vi "UDS Diagnostics Engine.vi"(8 "error in (no error)":errorcluster, 11 "State Variables":T1={"TCP Refs"={"Connection List"=refnum, "listener ID"=refnum}, "Stop"=refnum, "Top VI"=refnum, "Parameters"={"Properties"={"Name"="", "CAN"={"Database File"=path "", "CAN Interface"=enum."CAN0", "Baud Rate"=0, "Diagnostic Protocol"=enum."GMLAN", "Transport Protocol"=enum."ISO TP - Normal Mode", "Transmit ID"=0, "Receive ID"=0, "Transmit Extension"=0, "Receive Extension"=0, "Receive UUDT ID"=0, "Enable Stream"=TRUE, "VW TP Channel ID"=0, "Security"={"Source DLL Path"=path "", "Security Level"=1, "Target DLL Path"=path ""}, "Fill Frame"=FALSE, "Fill Byte"=255, "Termination"=FALSE}, "FPGA Settings"={"RT Bitfile Path"=path "", "RIO Device"=0, "Enable"=FALSE}, "PIDs"=[], "PID Lookup"=variant, "CPIDs"=[], "CPID Lookup"=variant, "DIDs"=[], "DID Lookup"=variant, "DPIDs"=[], "DPID Lookup"=variant, "DTC descriptor"={"DTC Byte Length"=2, "Status Byte Length"=1, "Add Data Byte Length"=1, "Byte Order"=enum."Motorola"}, "Routines"=[], "Routine Lookups"={"Start.Cmd"=variant, "Start.Resp"=variant, "Status.Cmd"=variant, "Status.Resp"=variant, "Stop.Cmd"=variant, "Stop.Resp"=variant}, "IO Control"=[], "IO.Cmd Lookup"=variant, "IO.Resp Lookup"=variant, "Memory Writes"=[], "Memory.Write Lookup"=variant, "Memory Reads"=[], "Memory.Read Lookup"=variant, "DTCControl"={"Description"="", "Signals"=[]}}, "ChanRefs"={"ToVS.PIDs"={"Name"="", "Write to VS Engine FIFO"=refnum, "Pairs"={"Refs"=[], "Values"=[]}}, "ToVS.DIDs"={"Name"="", "Write to VS Engine FIFO"=refnum, "Pairs"={"Refs"=[], "Values"=[]}}, "ToVS.DTCs"={"Name"="", "Write to VS Engine FIFO"=refnum, "Pairs"={"Refs"=[], "Values"=[]}}, "ToVS.DTCCount"={"Name"="", "Write to VS Engine FIFO"=refnum, "Pairs"={"Refs"=[], "Values"=[]}}, "ToVS.Status"={"Name"="", "Write to VS Engine FIFO"=refnum, "Pairs"={"Refs"=[], "Values"=[]}}, "FromVS.CPIDs"={"Name"="", "Read from VS Engine FIFO"=refnum, "Pairs"={"Refs"=[], "Values"=[]}}, "Cmds"={"Name"="", "Write to VS Engine FIFO"=refnum, "Read from VS Engine FIFO"=refnum, "Pairs"={"Chan Refs"=[], "Prev. Values"=[]}}, "FromVS.Routine.Start"={"Name"="", "Read from VS Engine FIFO"=refnum, "Pairs"={"Refs"=[], "Values"=[]}}, "ToVS.Routine.Start"={"Name"="", "Write to VS Engine FIFO"=refnum, "Pairs"={"Refs"=[], "Values"=[]}}, "FromVS.Routine.Status"={"Name"="", "Read from VS Engine FIFO"=refnum, "Pairs"={"Refs"=[], "Values"=[]}}, "ToVS.Routine.Status"={"Name"="", "Write to VS Engine FIFO"=refnum, "Pairs"={"Refs"=[], "Values"=[]}}, "FromVS.Routine.Stop"={"Name"="", "Read from VS Engine FIFO"=refnum, "Pairs"={"Refs"=[], "Values"=[]}}, "ToVS.Routine.Stop"={"Name"="", "Write to VS Engine FIFO"=refnum, "Pairs"={"Refs"=[], "Values"=[]}}, "FromVS.IO.Cmd"={"Name"="", "Read from VS Engine FIFO"=refnum, "Pairs"={"Refs"=[], "Values"=[]}}, "ToVS.IO.Resp"={"Name"="", "Write to VS Engine FIFO"=refnum, "Pairs"={"Refs"=[], "Values"=[]}}, "FromVS.WriteMemory"={"Name"="", "Read from VS Engine FIFO"=refnum, "Pairs"={"Refs"=[], "Values"=[]}}, "ToVS.ReadMemory"={"Name"="", "Write to VS Engine FIFO"=refnum, "Pairs"={"Refs"=[], "Values"=[]}}, "FromVS.DTCControl"={"Name"="", "Read from VS Engine FIFO"=refnum, "Pairs"={"Refs"=[], "Values"=[]}}}}, "ADCS Connection"={"Diag CAN Handle"=0, "Transport Protocol"=enum."ISO TP - Normal Mode", "Receive Address Extension"=0, "Transmit Address Extension"=0, "Receive CAN Id"=0, "Transmit CAN Id"=0, "Diag CAN Queue"=refnum, "Log Frames ?"=FALSE, "My TP Address"=0, "Other TP Address"=0, "T1"=0, "T2"=0, "T3"=0, "T4"=0, "Tx SN"=0, "Block Size"=0, "Rx SN"=0, "VW TP Initialized?"=FALSE, "Tx block no"=0, "baud rate"=0, "Interface"="", "Channel Diag CAN Handle"=0, "UDP Connection ID"=refnum, "TCP Connection ID"=refnum, "Target IP Addr"=0, "Source Address"=0, "Target Address"=0, "Send Header NACK?"=FALSE, "DLL Handle"=0, "NAD"=0, "Time Stamp read first"=0.0, "Time Stamp read last"=0.0, "Time Stamp write first"=0.0, "Time Stamp write last"=0.0, "Time Stamp write"=0.0, "Time Stamp read"=0.0}, "XNET References"={"Database"="", "GMLAN DPID Session"="", "Cluster"=""}, "BufferedCmds"=refnum, "XNETEngine (GMLAN)"=refnum} {"Parameters"."ChanRefs"."ToVS.ReadMemory"."Pairs"."Refs" format="%.0x"; "Parameters"."ChanRefs"."ToVS.IO.Resp"."Pairs"."Refs" format="%.0x"; "Parameters"."ChanRefs"."ToVS.Routine.Status"."Pairs"."Refs" format="%.0x"; "Parameters"."ChanRefs"."ToVS.Routine.Stop"."Pairs"."Refs" format="%.0x"; "Parameters"."ChanRefs"."ToVS.Routine.Start"."Pairs"."Refs" format="%.0x"; "Parameters"."ChanRefs"."Cmds"."Pairs"."Chan Refs" format="%.0x"; "Parameters"."ChanRefs"."ToVS.Status"."Pairs"."Refs" format="%.0x"; "Parameters"."ChanRefs"."ToVS.DTCCount"."Pairs"."Refs" format="%.0x"; "Parameters"."ChanRefs"."ToVS.DTCs"."Pairs"."Refs" format="%.0x"; "Parameters"."ChanRefs"."ToVS.PIDs"."Pairs"."Refs" format="%.0x"; "Parameters"."ChanRefs"."ToVS.DIDs"."Pairs"."Refs" format="%.0x"; "Parameters"."Properties"."DTCControl"."Signals"."Byte Order" items=["Little Endian", "Big Endian"]; "Parameters"."Properties"."DTCControl"."Signals"."Data Type" items=["Signed", "Unsigned", "IEEE Float"]; "Parameters"."Properties"."Memory Reads"."Signals"."Byte Order" items=["Little Endian", "Big Endian"]; "Parameters"."Properties"."Memory Reads"."Signals"."Data Type" items=["Signed", "Unsigned", "IEEE Float"]; "Parameters"."Properties"."Memory Writes"."Signals"."Byte Order" items=["Little Endian", "Big Endian"]; "Parameters"."Properties"."Memory Writes"."Signals"."Data Type" items=["Signed", "Unsigned", "IEEE Float"]; "Parameters"."Properties"."CPIDs"."Signals"."Byte Order" items=["Little Endian", "Big Endian"]; "Parameters"."Properties"."CPIDs"."Signals"."Data Type" items=["Signed", "Unsigned", "IEEE Float"]; "Parameters"."Properties"."DIDs"."Signals"."Byte Order" items=["Little Endian", "Big Endian"]; "Parameters"."Properties"."DIDs"."Signals"."Data Type" items=["Signed", "Unsigned", "IEEE Float"]; "Parameters"."Properties"."CAN"."Fill Byte" format="%.0x"; "Parameters"."Properties"."CAN"."VW TP Channel ID" format="%.0x"; "Parameters"."Properties"."CAN"."Receive UUDT ID" format="%.0x"; "Parameters"."Properties"."CAN"."Receive Extension" format="%.0x"; "Parameters"."Properties"."CAN"."Transmit Extension" format="%.0x"; "Parameters"."Properties"."CAN"."Receive ID" format="%.0x"; "Parameters"."Properties"."CAN"."Transmit ID" format="%.0x"; "Parameters"."Properties"."PIDs"."Signals"."Byte Order" items=["Little Endian", "Big Endian"]; "Parameters"."Properties"."PIDs"."Signals"."Data Type" items=["Signed", "Unsigned", "IEEE Float"]}) -> (0 "error out":errorcluster)   [LabVIEW 2015, in "Diagnostics Addon Engine.lvlib"]
doc: "Async loop that handles the UDS commands sent either by the channel engine or the TCP engine"
uses:
  Diagnostics Addon Engine.lvlib
  Stop FG/Stop Global Commands.ctl
  Stop FG/Stop FG.lvlib
  Error Handling API/Error Handling API.lvlib
  <vilib>/NI Veristand/Custom Device Tools/Custom Device Utility Library/Custom Device Utility Library.lvlib
  Shared/SubVIs/GUID Lookup.vi
  Shared/Diagnostics Addon Shared.lvlib
  Shared/Types/DTC and Timestamp Cluster.ctl
  Shared/Types/Datatable Lookup Positions.ctl
  <vilib>/NI/AMC/AMC.lvlib
  <vilib>/NI/Tools/Keyed Array/Tools_KeyedArray.lvlib
  GMLAN/GMLAN.lvlib
  GMLAN/_SubVIs/InitiateDiagnosticOperation_Parameter.ctl
  GMLAN/_SubVIs/InitiateDiagnosticOperation_SubFunctions.ctl
  GMLAN/_SubVIs/DisableNormalCommunication_Parameter.ctl
  GMLAN/_SubVIs/ReadDataByPacketIdentifier_SubFunctions.ctl
  <vilib>/Automotive Diagnostic Command Set/Diagnostic Transport.llb/Property ID.ctl
  <vilib>/addons/Automotive Diagnostic Command Set/NI_Automotive Diagnostic Command Set.lvlib
  Types/PID Data.ctl
  Shared/Types/ReadDTCbyDTCNumber Parameters.ctl
  GMLAN/_SubVIs/ReadFailureRecordData_readFailureRecordParameters_failureRecordIdentifier.ctl
  <vilib>/xnet/xnet.llb/XNET Convert (Signal to Frame Raw).vi
  <vilib>/xnet/xnet.llb/XNET Convert (Frame Raw to Signal).vi
  Shared/Types/Input Output Cmd Parameters.ctl
  STM/STM Lookup Table Ref.ctl
  Types/TCP Refs.ctl
  Shared/Types/Signal Parameters.ctl
  Shared/Types/Frame Parameters.ctl
  <vilib>/Automotive Diagnostic Command Set/Diagnostic Protocols.llb/DTC Descriptor.ctl
  Shared/Types/DPID Periodic Rate.ctl
  Shared/Types/DPID Parameters.ctl
  Shared/Types/Diagnostic Protocols.ctl
  Shared/Types/CAN Interface.ctl
  Shared/Types/CAN Configuration.ctl
  Shared/Types/Section Properties.ctl
  Types/Main Configuration.ctl
  Types/XNET References.ctl
  Types/State Variables.ctl
  <vilib>/NI Veristand/Custom Device API/Data Reference.ctl
  <vilib>/NI Veristand/Custom Device API/Custom Device API.lvlib
  Types/VS Data Channels.ctl
  <vilib>/NI Veristand/Custom Device API/Block Data Reference.ctl
  <vilib>/NI/Tools/Keyed Array/KeyedArray.ctl
  <vilib>/NI/AMC/Message.ctl
  <vilib>/NI/AMC/Message Queue.ctl
  Shared/Types/Transport Protocols.ctl
  <vilib>/Automotive Diagnostic Command Set/Diagnostic Transport.llb/Transport Protocol Selector.ctl
  <vilib>/Automotive Diagnostic Command Set/Diagnostic Transport.llb/Diag CAN Frame Log.ctl
  <vilib>/Automotive Diagnostic Command Set/Diagnostic Transport.llb/Diag Reference.ctl
  Inline Async API/Controls/Write To VS Engine.ctl
  Inline Async API/Inline Async API.lvlib
  Inline Async API/Controls/Read From VS Engine.ctl
  Inline Async API/Controls/ReadWrite Data.ctl
  Stop FG/Stop Global Ref.ctl
  Shared/Types/Security.ctl
  Shared/Types/FPGA Bitfile Settings.ctl
  Shared/Types/Command Response Signals.ctl
  Shared/Types/Routine Paramaters.ctl
  Shared/Types/IO Control Parameters.ctl
  Shared/Types/Compiled Routine Lookups.ctl
  Shared/Types/Exported DTC Control Cluster.ctl
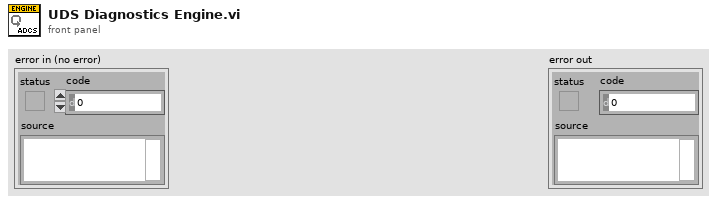
[diagram p1: front panel]
types:
  T1 = typedef "Diagnostics Addon Engine.lvlib/State Variables.ctl" = cluster{"TCP Refs":T2, "Stop":T4, "Top VI":refnum<vi>, "Parameters":T5, "ADCS Connection":T29, "XNET References":T31, "BufferedCmds":T32, "XNETEngine (GMLAN)":T32}
  T2 = typedef "Diagnostics Addon Engine.lvlib/TCP Refs.ctl" = cluster{"Connection List":T3, "listener ID":refnum<k5>}
  T3 = typedef "Diagnostics Addon Engine.lvlib/STM Lookup Table Ref.ctl" = refnum<vi>
  T4 = typedef "Diagnostics Addon Engine.lvlib/Stop FG.lvlib/Stop Global Ref.ctl" = refnum<vi>
  T5 = typedef "Diagnostics Addon Engine.lvlib/Main Configuration.ctl" = cluster{"Properties":T6, "ChanRefs":T23}
  T6 = typedef "Diagnostics Addon Shared.lvlib/Section Properties.ctl" = cluster{"Name":string, "CAN":T7, "FPGA Settings":T12, "PIDs":T13[], "PID Lookup":variant, "CPIDs":T13[], "CPID Lookup":variant, "DIDs":T13[], "DID Lookup":variant, "DPIDs":T15[], "DPID Lookup":variant, "DTC descriptor":T17, "Routines":T18[], "Routine Lookups":T20, "IO Control":T21[], "IO.Cmd Lookup":variant, "IO.Resp Lookup":variant, "Memory Writes":T13[], "Memory.Write Lookup":variant, "Memory Reads":T13[], "Memory.Read Lookup":variant, "DTCControl":T22}
  T7 = typedef "Diagnostics Addon Shared.lvlib/CAN Configuration.ctl" = cluster{"Database File":path, "CAN Interface":T8, "Baud Rate":u32, "Diagnostic Protocol":T9, "Transport Protocol":T10, "Transmit ID":u32, "Receive ID":u32, "Transmit Extension":u8, "Receive Extension":u8, "Receive UUDT ID":u32, "Enable Stream":bool, "VW TP Channel ID":u32, "Security":T11, "Fill Frame":bool, "Fill Byte":u8, "Termination":bool}
  T8 = typedef "Diagnostics Addon Shared.lvlib/CAN Interface.ctl" = enum16{"CAN0", "CAN1", "CAN2", "CAN3", "CAN4", "CAN5", "CAN6", "CAN7", "CAN8", "CAN9", "CAN10", "CAN11", "CAN12", "CAN13", "CAN14", "CAN15", "CAN16", "CAN17", "CAN18", "CAN19", "CAN20", "CAN21", "CAN22", "CAN23", "CAN24", "CAN25", "CAN26", "CAN27", "CAN28", "CAN29", "CAN30", "CAN31", "CAN32", "CAN33", "CAN34", "CAN35", "CAN36", "CAN37", "CAN38", "CAN39", "CAN40", "CAN41", "CAN42", "CAN43", "CAN44", "CAN45", "CAN46", "CAN47", "CAN48", "CAN49", "CAN50", "CAN51", "CAN52", "CAN53", "CAN54", "CAN55", "CAN56", "CAN57", "CAN58", "CAN59", "CAN60", "CAN61", "CAN62", "CAN63", "CAN 256 (Virtual)", "CAN 257 (Virtual)"}
  T9 = typedef "Diagnostics Addon Shared.lvlib/Diagnostic Protocols.ctl" = enum16{"GMLAN", "KWP-2000", "UDS"}
  T10 = typedef "Diagnostics Addon Shared.lvlib/Transport Protocols.ctl" = enum16{"ISO TP - Normal Mode", "ISO TP - Mixed Mode", "VW TP 2.0", "Diagnostics on IP"}
  T11 = typedef "Diagnostics Addon Shared.lvlib/Security.ctl" = cluster{"Source DLL Path":path, "Security Level":u8, "Target DLL Path":path}
  T12 = typedef "Diagnostics Addon Shared.lvlib/FPGA Bitfile Settings.ctl" = cluster{"RT Bitfile Path":path, "RIO Device":u16, "Enable":bool}
  T13 = typedef "Diagnostics Addon Shared.lvlib/Frame Parameters.ctl" = cluster{"Name":string, "Description":string, "ID":u32, "Signals":T14[]}
  T14 = typedef "Diagnostics Addon Shared.lvlib/Signal Parameters.ctl" = cluster{"Start Bit":u8, "Length":u8, "Scaling Factor":dbl, "Scaling Offset":dbl, "Minimum":dbl, "Maximum":dbl, "Data Type":u32, "Byte Order":u32, "Default Value":dbl, "Name":string, "Units":string, "Description":string}
  T15 = typedef "Diagnostics Addon Shared.lvlib/DPID Parameters.ctl" = cluster{"DPID ID":u8, "Speed":T16, "PIDs":u16[]}
  T16 = typedef "Diagnostics Addon Shared.lvlib/DPID Periodic Rate.ctl" = enum16{"Slow", "Medium", "Fast"}
  T17 = typedef "Diagnostics Addon Shared.lvlib/DTC Descriptor.ctl" = cluster{"DTC Byte Length":i32, "Status Byte Length":i32, "Add Data Byte Length":i32, "Byte Order":enum16{"Motorola", "Intel"}}
  T18 = typedef "Diagnostics Addon Shared.lvlib/Routine Paramaters.ctl" = cluster{"Name":string, "Description":string, "ID":u16, "Start Parameters":T19, "Request Parameters":T19, "Stop Parameters":T19}
  T19 = typedef "Diagnostics Addon Shared.lvlib/Command Response Signals.ctl" = cluster{"Cmd":T14[], "Response":T14[]}
  T20 = typedef "Diagnostics Addon Shared.lvlib/Compiled Routine Lookups.ctl" = cluster{"Start.Cmd":variant, "Start.Resp":variant, "Status.Cmd":variant, "Status.Resp":variant, "Stop.Cmd":variant, "Stop.Resp":variant}
  T21 = typedef "Diagnostics Addon Shared.lvlib/IO Control Parameters.ctl" = cluster{"Name":string, "Description":string, "ID":u16, "Signals":T19}
  T22 = typedef "Diagnostics Addon Shared.lvlib/Exported DTC Control Cluster.ctl" = cluster{"Description":string, "Signals":T14[]}
  T23 = typedef "Diagnostics Addon Engine.lvlib/VS Data Channels.ctl" = cluster{"ToVS.PIDs":T24, "ToVS.DIDs":T24, "ToVS.DTCs":T24, "ToVS.DTCCount":T24, "ToVS.Status":T24, "FromVS.CPIDs":T26, "Cmds":T28, "FromVS.Routine.Start":T26, "ToVS.Routine.Start":T24, "FromVS.Routine.Status":T26, "ToVS.Routine.Status":T24, "FromVS.Routine.Stop":T26, "ToVS.Routine.Stop":T24, "FromVS.IO.Cmd":T26, "ToVS.IO.Resp":T24, "FromVS.WriteMemory":T26, "ToVS.ReadMemory":T24, "FromVS.DTCControl":T26}
  T24 = typedef "Diagnostics Addon Engine.lvlib/Inline Async API.lvlib/Write To VS Engine.ctl" = cluster{"Name":string, "Write to VS Engine FIFO":refnum<k33>, "Pairs":cluster{"Refs":T25[], "Values":dbl[]}}
  T25 = typedef "Custom Device API.lvlib/Data Reference.ctl" = i32
  T26 = typedef "Diagnostics Addon Engine.lvlib/Inline Async API.lvlib/Read From VS Engine.ctl" = cluster{"Name":string, "Read from VS Engine FIFO":refnum<k33>, "Pairs":cluster{"Refs":T27[], "Values":dbl[]}}
  T27 = typedef "Custom Device API.lvlib/Block Data Reference.ctl" = cluster{"Data Reference":T25, "Offset":u64, "Length":u64}
  T28 = typedef "Diagnostics Addon Engine.lvlib/Inline Async API.lvlib/ReadWrite Data.ctl" = cluster{"Name":string, "Write to VS Engine FIFO":refnum<k33>, "Read from VS Engine FIFO":refnum<k33>, "Pairs":cluster{"Chan Refs":T25[], "Prev. Values":dbl[]}}
  T29 = typedef "NI_Automotive Diagnostic Command Set.lvlib/Diag Reference.ctl" = cluster{"Diag CAN Handle":u32, "Transport Protocol":T30, "Receive Address Extension":u8, "Transmit Address Extension":u8, "Receive CAN Id":u32, "Transmit CAN Id":u32, "Diag CAN Queue":refnum<queue>, "Log Frames ?":bool, "My TP Address":u8, "Other TP Address":u8, "T1":u16, "T2":u16, "T3":u16, "T4":u16, "Tx SN":u8, "Block Size":u8, "Rx SN":u8, "VW TP Initialized?":bool, "Tx block no":u8, "baud rate":u32, "Interface":string, "Channel Diag CAN Handle":u32, "UDP Connection ID":refnum<k16>, "TCP Connection ID":refnum<k5>, "Target IP Addr":u32, "Source Address":u16, "Target Address":u16, "Send Header NACK?":bool, "DLL Handle":u32, "NAD":u8, "Time Stamp read first":dbl, "Time Stamp read last":dbl, "Time Stamp write first":dbl, "Time Stamp write last":dbl, "Time Stamp write":dbl, "Time Stamp read":dbl}
  T30 = typedef "NI_Automotive Diagnostic Command Set.lvlib/Transport Protocol Selector.ctl" = enum16{"ISO TP - Normal Mode", "ISO TP - Mixed Mode", "VW TP 2.0", "Diagnostics on IP", "ISO TP LIN"}
  T31 = typedef "Diagnostics Addon Engine.lvlib/XNET References.ctl" = cluster{"Database":refnum<k21>, "GMLAN DPID Session":refnum<k21>, "Cluster":refnum<k21>}
  T32 = typedef "AMC.lvlib/Message Queue.ctl" = refnum<queue>
  T33 = typedef "Diagnostics Addon Shared.lvlib/DTC and Timestamp Cluster.ctl" = cluster{"Timestamp":dbl, "DTC":dbl, "Status":dbl, "Add Data":dbl}
  T34 = typedef "Diagnostics Addon Engine.lvlib/Stop FG.lvlib/Stop Global Commands.ctl" = enum16{"Write", "Read", "Reset"}
  T35 = typedef "NI_Automotive Diagnostic Command Set.lvlib/Property ID.ctl" = enum16{"Timeout Diag Command", "Timeout FC (Bs)", "Timeout CF (Cr)", "Receive Block Size (BS)", "Wait Time CF (STmin)", "Max Wait Frames (N_WFTmax)", "Wait Frames to Send (N_WAIT)", "Time between Waits (T_W)", "Fill CAN Frames", "Fill Byte", "Invalid Response as Error", "Max RspPending Count", "VWTP Command Timeout", "STmin", "P2min", "Termination"}
  T36 = typedef "Diagnostics Addon Shared.lvlib/ReadDTCbyDTCNumber Parameters.ctl" = cluster{"DTC":u16, "FailTypeByte":u8}
  T37 = typedef "GMLAN.lvlib/ReadFailureRecordData_readFailureRecordParameters_failureRecordIdentifier.ctl" = cluster{"failureRecordNumber":u8, "DTC ID":u16, "DTCFailureType":u8}
  T38 = enum16{"open", "replace", "create", "open or create", "replace or create", "replace or create with confirmation"}
  T39 = typedef "GMLAN.lvlib/ReadDataByPacketIdentifier_SubFunctions.ctl" = enum8{"stopSending", "sendOneResponse", "scheduleAtSlowRate", "scheduleAtMediumRate", "scheduleAtFastRate"}
  T40 = typedef "GMLAN.lvlib/InitiateDiagnosticOperation_Parameter.ctl" = enum8{"SpecificECU", "EntireNetwork"}
  T41 = typedef "GMLAN.lvlib/DisableNormalCommunication_Parameter.ctl" = enum8{"SpecificECU", "EntireNetwork"}
  T42 = typedef "Diagnostics Addon Engine.lvlib/PID Data.ctl" = cluster{"ID":u16, "Raw Frame":u8[]}
  T43 = cluster{"resp":u8[], "error code":u8, "error out":errorcluster}
  T44 = typedef "Diagnostics Addon Shared.lvlib/Datatable Lookup Positions.ctl" = cluster{"Offset":i32, "Length":i32, "ByteLength":u16}
  T45 = typedef "Diagnostics Addon Shared.lvlib/Input Output Cmd Parameters.ctl" = cluster{"ID":u16, "Mode":u8}
  T46 = typedef "AMC.lvlib/Message.ctl" = cluster{"name":string, "value":string, "attributes":T47, "receiver host":string, "receiver process":string, "source host":string, "source process":string, "priority message":bool, "acknowledge message":bool}
  T47 = typedef "Tools_KeyedArray.lvlib/KeyedArray.ctl" = cluster{"keys":string[], "values":string[]}
  T48 = cluster{"Boolean array[0]":bool, "Boolean array[1]":bool, "Boolean array[2]":bool, "Boolean array[3]":bool, "Boolean array[4]":bool, "Boolean array[5]":bool, "Boolean array[6]":bool, "Boolean array[7]":bool}
  T49 = typedef "Diagnostics Addon Engine.lvlib/Filtered DPID IDs.ctl" = cluster{"Slow":u8[], "Medium":u8[], "Fast":u8[]}
  T50 = typedef "GMLAN.lvlib/InitiateDiagnosticOperation_SubFunctions.ctl" = u8
  T51 = typedef "Diagnostic Trouble Code.ctl" = cluster{"DTC":u32, "Status":u32, "Add Data":u32}
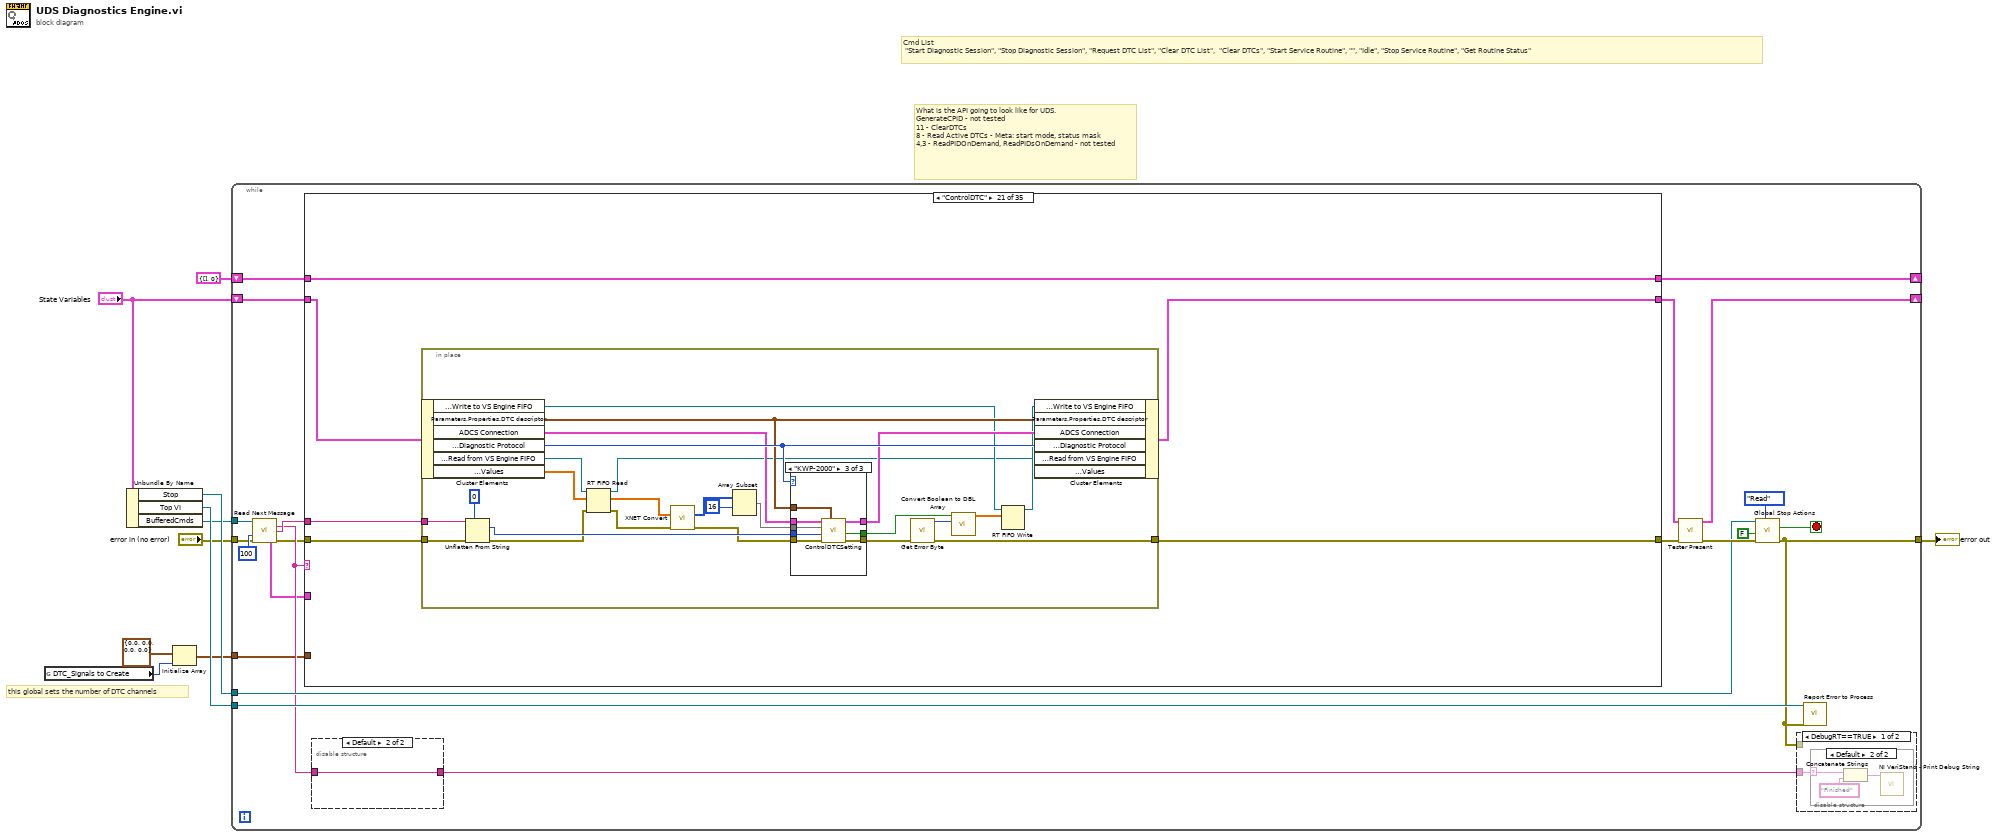
[diagram p0: block diagram]
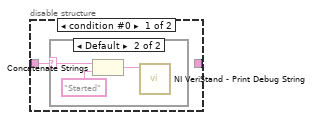
[diagram p2: hidden frame]
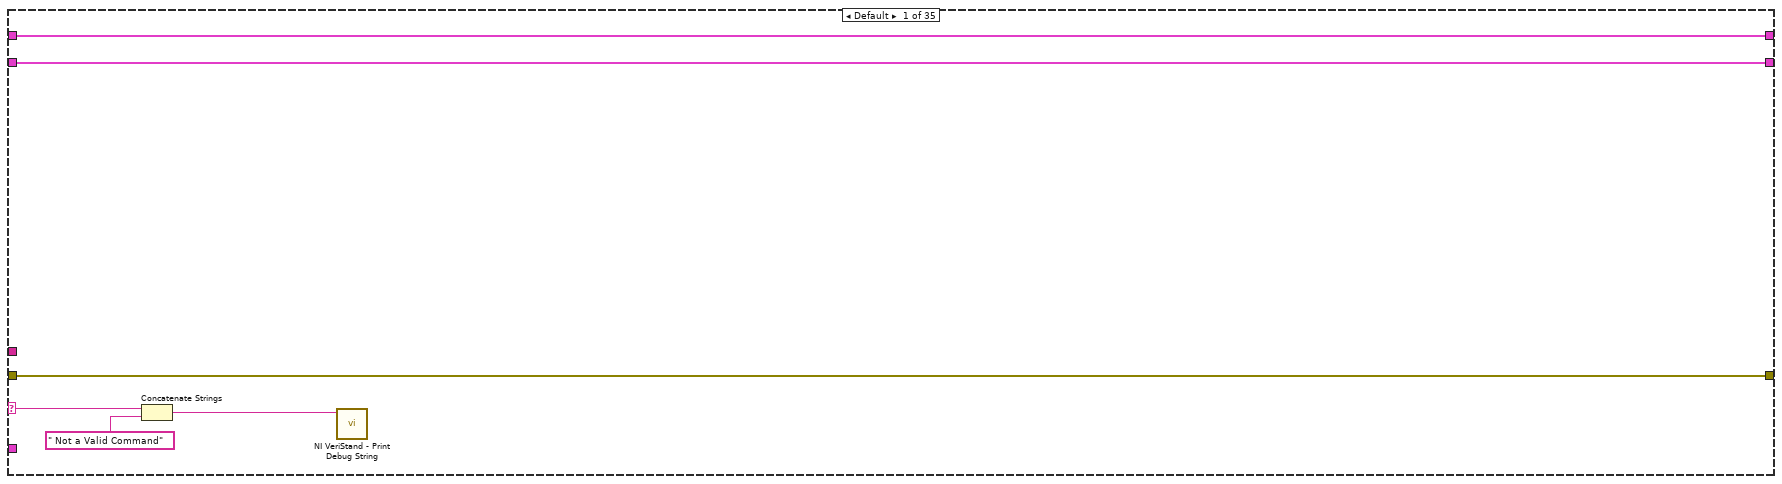
[diagram p6: hidden frame]
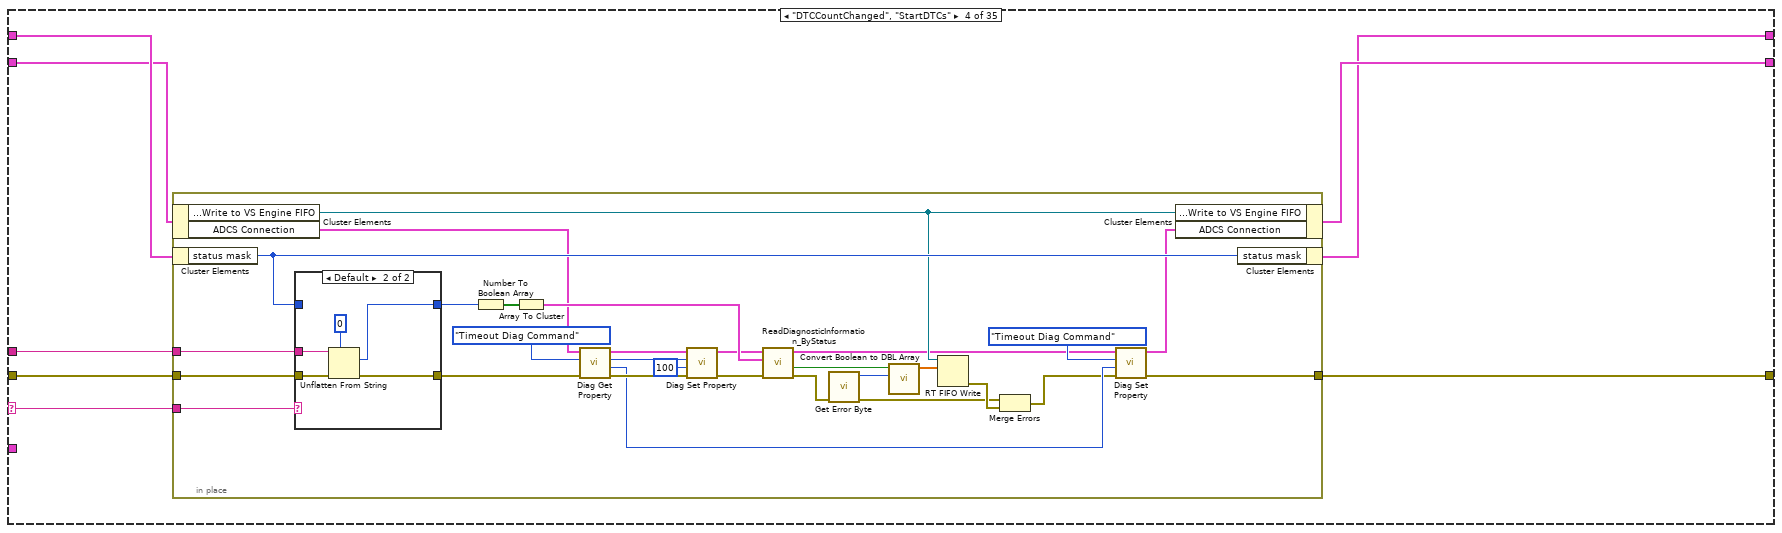
[diagram p9: hidden frame]
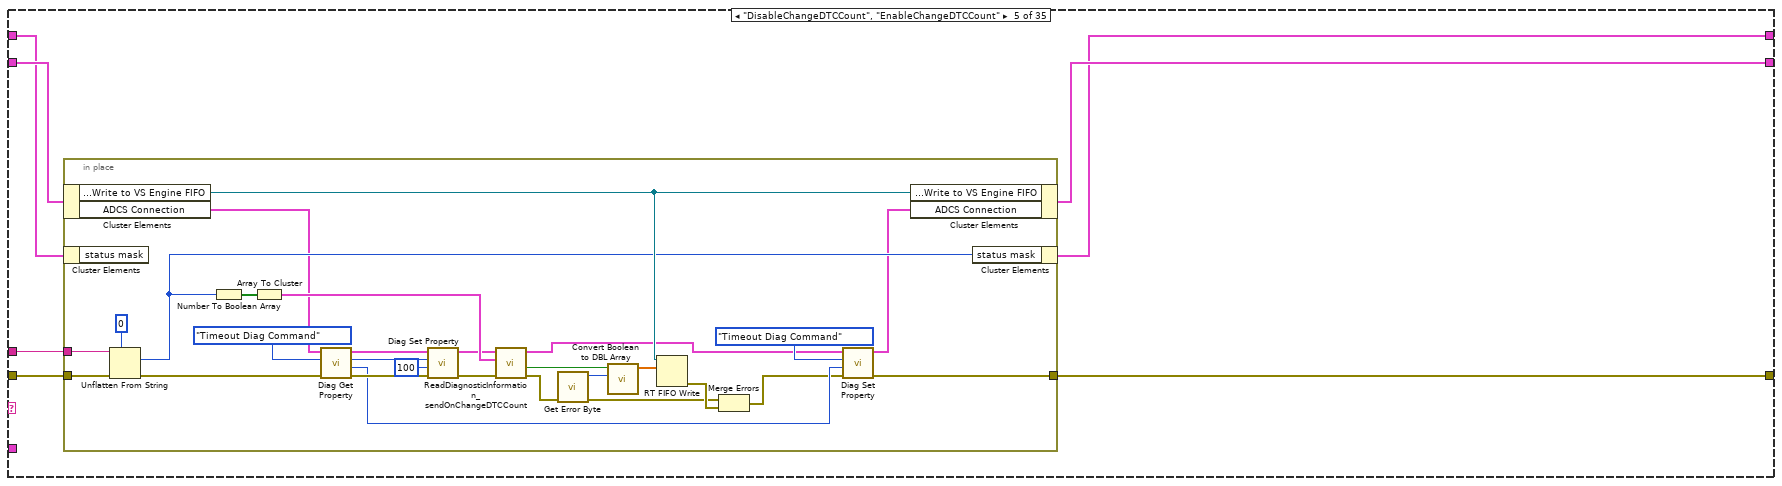
[diagram p11: hidden frame]
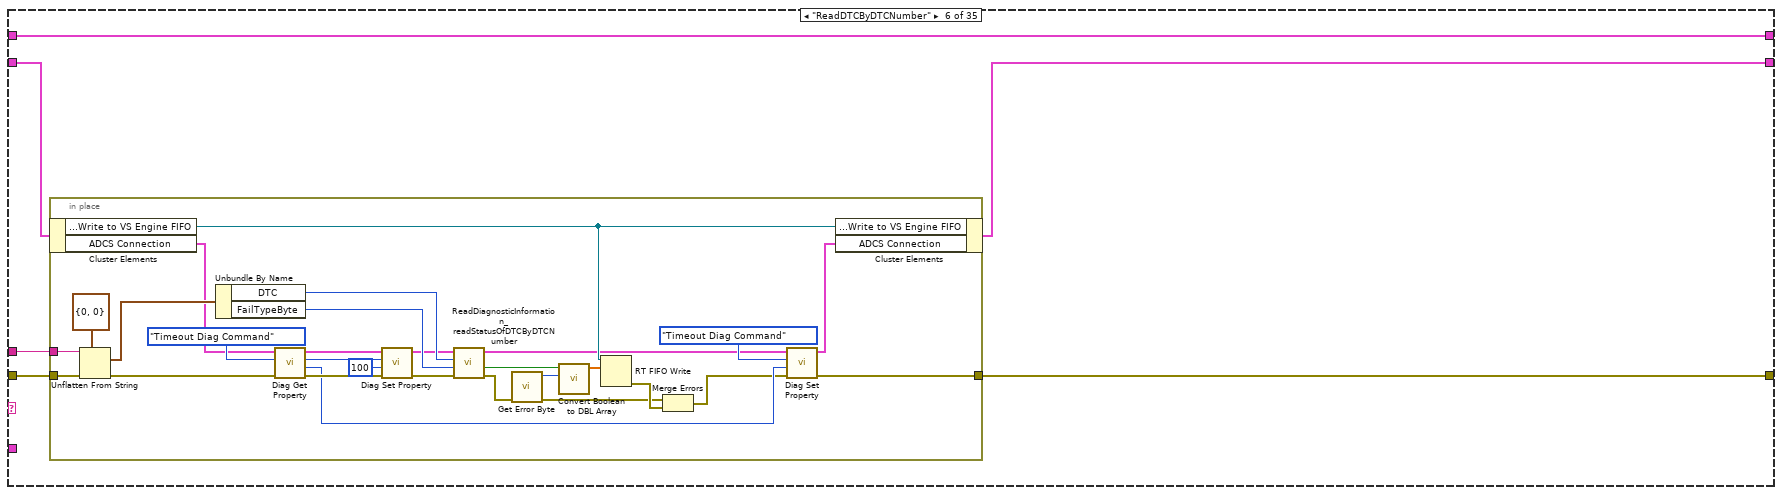
[diagram p12: hidden frame]
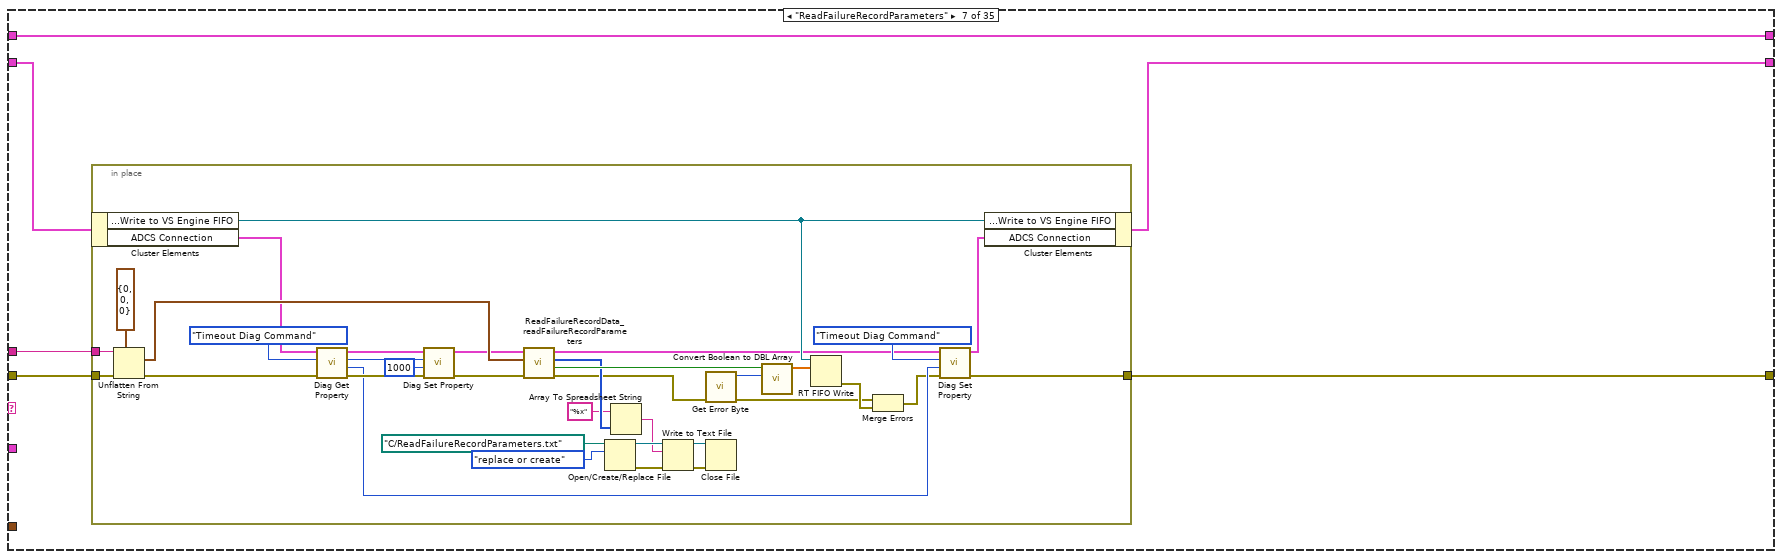
[diagram p13: hidden frame]
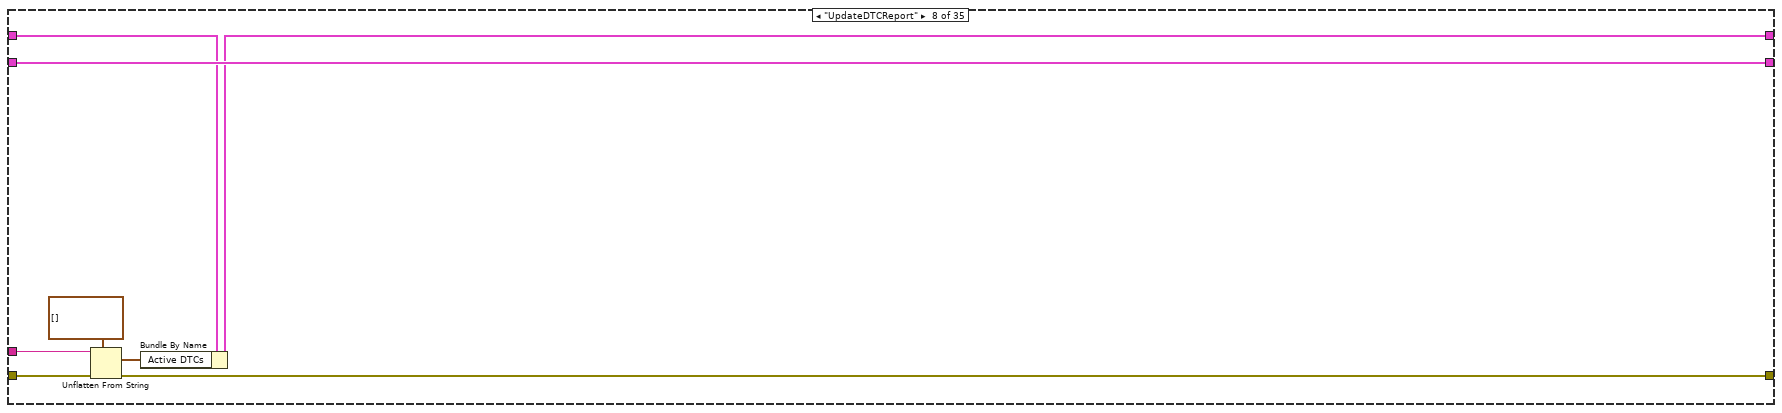
[diagram p14: hidden frame]
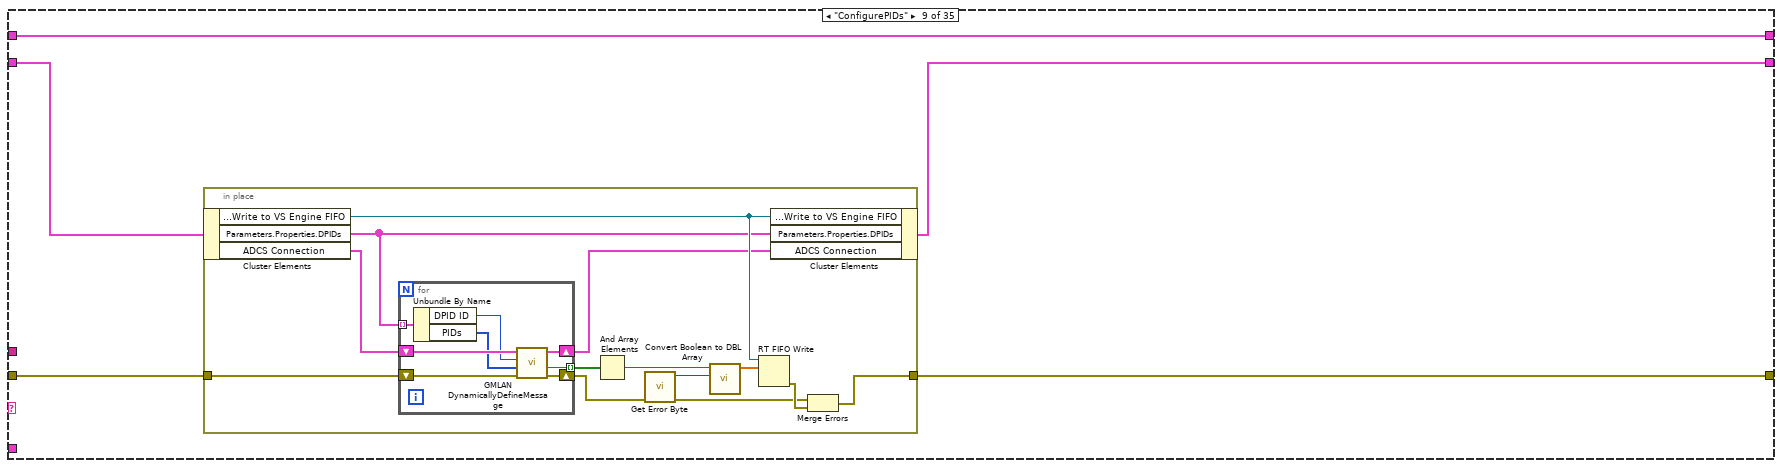
[diagram p15: hidden frame]
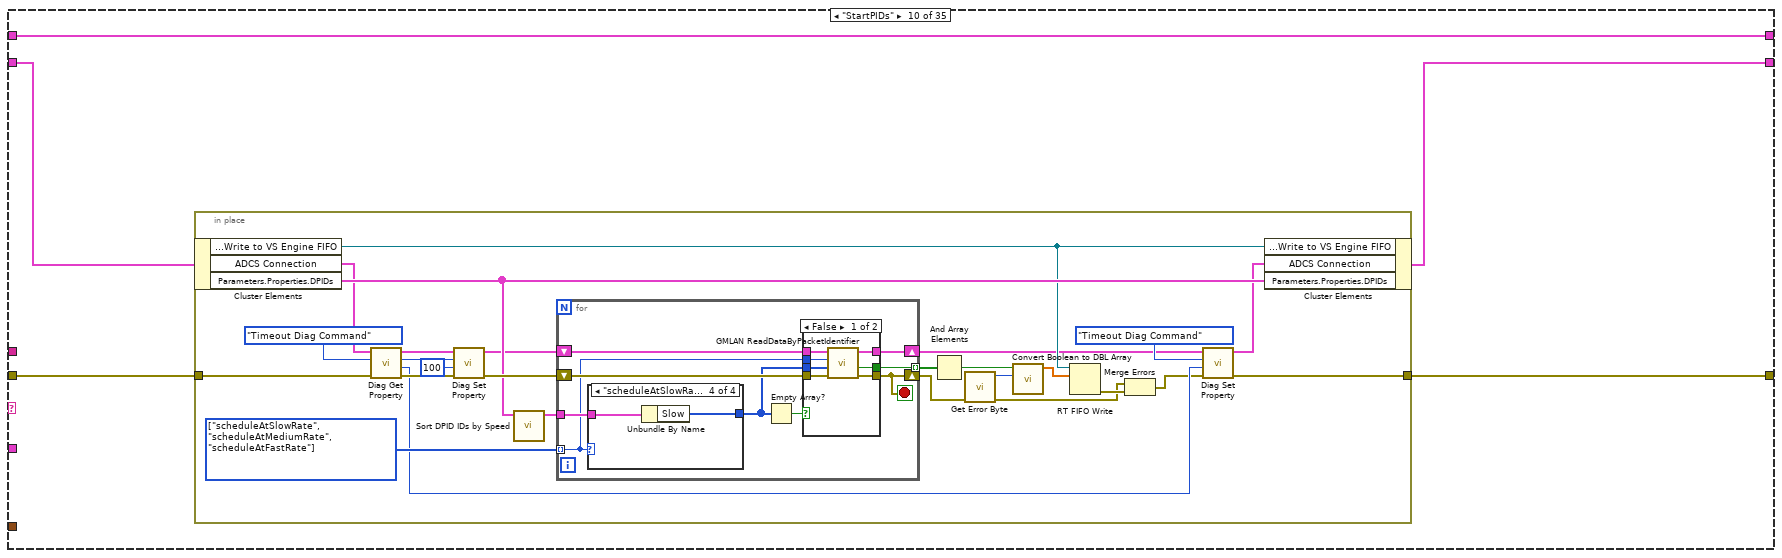
[diagram p16: hidden frame]
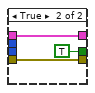
[diagram p17: hidden frame]
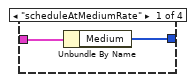
[diagram p18: hidden frame]
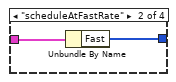
[diagram p19: hidden frame]
diagram:
  # "this global sets the number of DTC channels"
  # "What is the API going to look like for UDS.\nGenerateCPID - not tested\n11 - ClearDTCs\n8 - Read Active DTCs - Meta: start mode, status mask \n4,3 - ReadPIDOnDemand, ReadPIDsOnDemand - not tested"
  # "Cmd List\n \"Start Diagnostic Session\", \"Stop Diagnostic Session\", \"Request DTC List\", \"Clear DTC List\",  \"Clear DTCs\", \"Start Service Routine\", \"\", \"Idle\", \"Stop Service Routine\", \"Get Routine Status\""
  n1 = global read "GUID Lookup.vi" "DTC_Signals to Create"() -> (w3:i32)
  n2 = Unbundle By Name("State Variables") -> ("Stop"=w10:T4, "Top VI"=w9:refnum<vi>, "BufferedCmds"=w5:T32)
  n3 = Initialize Array(T33 {"Timestamp"=0.0, "DTC"=0.0, "Status"=0.0, "Add Data"=0.0} ("Diagnostic Trouble Code"), w3) -> (w2:T33[])
  n4 = while {
    tunnel: w5 -> [w32]
    tunnel: w9 -> [w24]
    tunnel: "error in (no error)" -> [w30]
    tunnel: [w11] -> w8
    tunnel: w10 -> [w23]
    shift-right: [w22] -> _
    shift-left: cluster{"Active DTCs":T33[], "status mask":u8} {"Active DTCs"=[], "status mask"=0} -> [w21]
    tunnel: w2 -> [w18]
    shift-right: [w15] -> _
    shift-left: "State Variables" -> [w17]
    stop <- w25 stop-if-true
    n5 = call <vilib>:"Read Next Message.vi"("message queue in"=w32, "timeout (1 ms)"=100 ("timeout (1ms)"), "error in"=w30) -> ("message name"=w20:string, "message value"=w29:string, "message"=w19:T46, "error out"=w14:errorcluster)  [unwired: 5 in, 4 out]
    n6 = case shown="\"ControlDTC\"" w20 {
      selector: w20 -> [w43 _ _ w59 _ _ _ _ _ _ _ _ _ _ _ _ _ _ _ _ _ w762 _ w971 w1058 _ _ w1149 _ _ _ _ _ _ _]
      tunnel: w14 -> [w47 w50 w51 w61 w103 w134 w167 w208 w215 w239 w296 w335 w338 w344 w358 w398 w434 w471 w508 w530 w711 w759 w870 w973 w1057 w1108 w1142 w1147 w1185 w1192 w1245 w1294 w1419 w1478 w1535]
      tunnel: w29 -> [_ _ _ w58 w101 w135 w168 w204 _ _ _ _ _ _ w356 _ _ _ _ w529 w709 w760 w869 w972 w1056 w1106 _ w1148 _ w1190 w1243 w1293 w1415 w1477 w1534]
      tunnel: [w47 w50 w51 w60 w102 w133 w166 w207 w214 w238 w295 w335 w338 w343 w357 w399 w435 w472 w507 w532 w710 w761 w868 w970 w1055 w1107 w1142 w1150 w1185 w1191 w1244 w1292 w1418 w1476 w1532] -> w12
      tunnel: [w46 w49 w53 w54 w97 w136 w169 w205 w216 w242 w297 w337 w340 w345 w359 w400 w436 w473 w509 w525 w714 _ w871 w974 w1059 w1109 w1144 w1152 w1187 w1193 w1246 w1295 w1420 w1479 w1537] -> w22
      tunnel: w21 -> [w46 w49 w53 w57 w98 w136 w169 w206 w216 w242 w297 w337 w340 w345 w359 w400 w436 w473 w509 w526 w714 _ w871 w974 w1059 w1109 w1144 w1152 w1187 w1193 w1246 w1295 w1420 w1479 w1537]
      tunnel: w19 -> [_ _ _ _ _ _ _ _ _ _ _ _ _ _ _ _ _ _ _ w531 _ w763 _ _ _ _ _ w1151 _ _ _ _ _ _ _]
      tunnel: w18 -> [_ _ _ _ _ _ _ _ _ _ _ _ _ _ _ _ _ _ _ w528 _ _ _ _ _ _ _ _ _ _ _ _ _ _ _]
      tunnel: w17 -> [w42 w48 w52 w56 w100 w132 w165 w211 w213 w241 w294 w336 w339 w342 w355 w397 w433 w470 w506 w527 w713 w758 w867 w969 w1054 w1105 w1143 w1146 w1186 w1189 w1242 w1291 w1417 w1475 w1536]
      tunnel: [w42 w48 w52 w55 w99 w131 w164 w211 w212 w240 w293 w336 w339 w341 w354 w396 w432 w469 w505 w524 w712 w757 w866 w968 w1053 w1104 w1143 w1145 w1186 w1188 w1241 w1290 w1416 w1474 w1533] -> w16
      frame Default {
        n7 = Concatenate Strings(w43, " Not a Valid Command" ("string")) -> (w44:string)
        n8 = call <vilib>:"NI VeriStand - Print Debug String.vi"("Message"=w44) -> ()  [unwired: 10 in, 1 out]
      }
      frame "" {
      }
      frame "<--------------- GMLAN ONLY --------------->" {
      }
      frame "DTCCountChanged", "StartDTCs" {
        n9 = in-place {
          in-place-border: w61 -> [w75]
          in-place-border: [w74] -> w60
          in-place-border: w59 -> [w73]
          in-place-border: w58 -> [w72]
          w87 = Property_ID."Timeout Diag Command" ("property ID")
          n10 = in-place-cluster #1(w56) -> ("Parameters.ChanRefs.ToVS.Status.Write to VS Engine FIFO"=w70:refnum<k33>, "ADCS Connection"=w68:T29)
          n11 = in-place-cluster #2(w57) -> ("status mask"=w71:u8)
          n12 = case shown="Default" w73 {
            tunnel: w75 -> [w91 w96]
            tunnel: w72 -> [_ w95]
            tunnel: [w90 w93] -> w78
            tunnel: [w91 w92] -> w85
            tunnel: w71 -> [w90 _]
            frame "DTCCountChanged" {
            }
            frame Default {
              n13 = Unflatten From String(type=u8 0 ("status mask"), binary string=w95, error in (no error)=w96) -> (value=w93:u8, error out=w92:errorcluster)  [unwired: 2 in, 1 out]
            }
          }
          n14 = Number To Boolean Array(number=w78) -> (Boolean array=w77:bool[])
          n15 = Array To Cluster(array=w77) -> (cluster=w76:T48)
          n16 = call <vilib>:"Diag Get Property.vi"("error in (no error)"=w85, "property ID"=w87, "diag ref in"=w68) -> ("error out"=w89:errorcluster, "property value"=w83:u32, "diag ref out"=w69:T29)  [unwired: 6 in]
          n17 = call <vilib>:"Diag Set Property.vi"("error in (no error)"=w89, "property value"=u32 100, "property ID"=w87, "diag ref in"=w69) -> ("error out"=w84:errorcluster, "diag ref out"=w67:T29)  [unwired: 6 in]
          n18 = call "ReadDiagnosticInformation_ByStatus.vi"("error in (no error)"=w84, "status mask"=w76, "diag ref in"=w67) -> ("error out"=w64:errorcluster, "success?"=w81:bool, "diag ref out"=w66:T29)  [unwired: 5 in, 1 out]
          n19 = call "Get Error Byte.vi"("error"=w64) -> ("error  out"=w63:errorcluster, "Error Byte"=w62:u8)  [unwired: 9 in]
          n20 = call "Convert Boolean to DBL Array.vi"("Error Code"=w62, "Boolean"=w81) -> ("DBL Array"=w82:dbl[])  [unwired: 9 in]
          n21 = RT FIFO Write(0:w70, 1:w82) -> (11:w80:errorcluster)  [unwired: 3 in, 3 out]
          n22 = Merge Errors(w63, w80) -> (w79:errorcluster)
          n23 = call <vilib>:"Diag Set Property.vi"("error in (no error)"=w79, "property value"=w83, "property ID"=Property_ID."Timeout Diag Command", "diag ref in"=w66) -> ("error out"=w74:errorcluster, "diag ref out"=w65:T29)  [unwired: 6 in]
          n24 = in-place-cluster #1("Parameters.ChanRefs.ToVS.Status.Write to VS Engine FIFO"=w70, "ADCS Connection"=w65) -> (w55:T1)
          n25 = in-place-cluster #2("status mask"=w71) -> (w54:cluster{"Active DTCs":T33[], "status mask":u8})
        }
      }
      frame "DisableChangeDTCCount", "EnableChangeDTCCount" {
        n26 = in-place {
          in-place-border: w103 -> [w116]
          in-place-border: [w115] -> w102
          in-place-border: w101 -> [w114]
          w127 = Property_ID."Timeout Diag Command" ("property ID")
          n27 = in-place-cluster #3(w100) -> ("Parameters.ChanRefs.ToVS.Status.Write to VS Engine FIFO"=w113:refnum<k33>, "ADCS Connection"=w110:T29)
          n28 = in-place-cluster #4(w98) -> ()  [unwired: 1 out]
          n29 = Unflatten From String(type=u8 0 ("status mask"), binary string=w114, error in (no error)=w116) -> (value=w112:u8, error out=w125:errorcluster)  [unwired: 2 in, 1 out]
          n30 = Number To Boolean Array(number=w112) -> (Boolean array=w118:bool[])
          n31 = Array To Cluster(array=w118) -> (cluster=w117:T48)
          n32 = call <vilib>:"Diag Get Property.vi"("error in (no error)"=w125, "property ID"=w127, "diag ref in"=w110) -> ("error out"=w129:errorcluster, "property value"=w123:u32, "diag ref out"=w111:T29)  [unwired: 6 in]
          n33 = call <vilib>:"Diag Set Property.vi"("error in (no error)"=w129, "property value"=u32 100, "property ID"=w127, "diag ref in"=w111) -> ("error out"=w124:errorcluster, "diag ref out"=w109:T29)  [unwired: 6 in]
          n34 = call "ReadDiagnosticInformation_sendOnChangeDTCCount.vi"("error in (no error)"=w124, "status mask"=w117, "diag ref in"=w109) -> ("error out"=w106:errorcluster, "success?"=w121:bool, "diag ref out"=w108:T29)  [unwired: 5 in, 1 out]
          n35 = call "Get Error Byte.vi"("error"=w106) -> ("error  out"=w105:errorcluster, "Error Byte"=w104:u8)  [unwired: 9 in]
          n36 = call "Convert Boolean to DBL Array.vi"("Error Code"=w104, "Boolean"=w121) -> ("DBL Array"=w122:dbl[])  [unwired: 9 in]
          n37 = RT FIFO Write(0:w113, 1:w122) -> (11:w120:errorcluster)  [unwired: 3 in, 3 out]
          n38 = Merge Errors(w105, w120) -> (w119:errorcluster)
          n39 = call <vilib>:"Diag Set Property.vi"("error in (no error)"=w119, "property value"=w123, "property ID"=Property_ID."Timeout Diag Command", "diag ref in"=w108) -> ("error out"=w115:errorcluster, "diag ref out"=w107:T29)  [unwired: 6 in]
          n40 = in-place-cluster #3("Parameters.ChanRefs.ToVS.Status.Write to VS Engine FIFO"=w113, "ADCS Connection"=w107) -> (w99:T1)
          n41 = in-place-cluster #4("status mask"=w112) -> (w97:cluster{"Active DTCs":T33[], "status mask":u8})
        }
      }
      frame "ReadDTCByDTCNumber" {
        n42 = in-place {
          in-place-border: w135 -> [w148]
          in-place-border: w134 -> [w147]
          in-place-border: [w145] -> w133
          w161 = Property_ID."Timeout Diag Command" ("property ID")
          n43 = in-place-cluster #5(w132) -> ("Parameters.ChanRefs.ToVS.Status.Write to VS Engine FIFO"=w146:refnum<k33>, "ADCS Connection"=w143:T29)
          n44 = Unflatten From String(type=T36 {"DTC"=0, "FailTypeByte"=0}, binary string=w148, error in (no error)=w147) -> (value=w151:T36, error out=w159:errorcluster)  [unwired: 2 in, 1 out]
          n45 = Unbundle By Name(w151) -> ("DTC"=w150:u16, "FailTypeByte"=w149:u8)
          n46 = call <vilib>:"Diag Get Property.vi"("error in (no error)"=w159, "property ID"=w161, "diag ref in"=w143) -> ("error out"=w163:errorcluster, "property value"=w157:u32, "diag ref out"=w144:T29)  [unwired: 6 in]
          n47 = call <vilib>:"Diag Set Property.vi"("error in (no error)"=w163, "property value"=u32 100, "property ID"=w161, "diag ref in"=w144) -> ("error out"=w158:errorcluster, "diag ref out"=w142:T29)  [unwired: 6 in]
          n48 = call "ReadDiagnosticInformation_readStatusOfDTCByDTCNumber.vi"("error in (no error)"=w158, "FailTypeByte"=w149, "DTC"=w150, "diag ref in"=w142) -> ("error out"=w139:errorcluster, "success?"=w155:bool, "diag ref out"=w141:T29)  [unwired: 4 in, 1 out]
          n49 = call "Get Error Byte.vi"("error"=w139) -> ("error  out"=w138:errorcluster, "Error Byte"=w137:u8)  [unwired: 9 in]
          n50 = call "Convert Boolean to DBL Array.vi"("Error Code"=w137, "Boolean"=w155) -> ("DBL Array"=w156:dbl[])  [unwired: 9 in]
          n51 = RT FIFO Write(0:w146, 1:w156) -> (11:w154:errorcluster)  [unwired: 3 in, 3 out]
          n52 = Merge Errors(w138, w154) -> (w153:errorcluster)
          n53 = call <vilib>:"Diag Set Property.vi"("error in (no error)"=w153, "property value"=w157, "property ID"=Property_ID."Timeout Diag Command", "diag ref in"=w141) -> ("error out"=w145:errorcluster, "diag ref out"=w140:T29)  [unwired: 6 in]
          n54 = in-place-cluster #5("Parameters.ChanRefs.ToVS.Status.Write to VS Engine FIFO"=w146, "ADCS Connection"=w140) -> (w131:T1)
        }
      }
      frame "ReadFailureRecordParameters" {
        n55 = in-place {
          in-place-border: w168 -> [w181]
          in-place-border: w167 -> [w180]
          in-place-border: [w179] -> w166
          w201 = Property_ID."Timeout Diag Command" ("property ID")
          n56 = in-place-cluster #6(w165) -> ("Parameters.ChanRefs.ToVS.Status.Write to VS Engine FIFO"=w178:refnum<k33>, "ADCS Connection"=w176:T29)
          n57 = Unflatten From String(type=T37 {"failureRecordNumber"=0, "DTC ID"=0, "DTCFailureType"=0} ("failureRecordIdentifier"), binary string=w181, error in (no error)=w180) -> (value=w182:T37, error out=w199:errorcluster)  [unwired: 2 in, 1 out]
          n58 = call <vilib>:"Diag Get Property.vi"("error in (no error)"=w199, "property ID"=w201, "diag ref in"=w176) -> ("error out"=w203:errorcluster, "property value"=w197:u32, "diag ref out"=w177:T29)  [unwired: 6 in]
          n59 = call <vilib>:"Diag Set Property.vi"("error in (no error)"=w203, "property value"=u32 1000, "property ID"=w201, "diag ref in"=w177) -> ("error out"=w198:errorcluster, "diag ref out"=w175:T29)  [unwired: 6 in]
          n60 = call "ReadFailureRecordData_readFailureRecordParameters.vi"("error in (no error)"=w198, "failureRecordIdentifier"=w182, "diag ref in"=w175) -> ("error out"=w172:errorcluster, "success?"=w195:bool, "data out"=w188:u8[], "diag ref out"=w174:T29)  [unwired: 5 in]
          n61 = Open/Create/Replace File(file path (use dialog)=path "C:/ReadFailureRecordParameters.txt", operation (0:open)=T38."replace or create") -> (refnum out=w186:refnum<file>, error out=w190:errorcluster)  [unwired: 4 in, 1 out]
          n62 = Array To Spreadsheet String(array=w188, 3:"%x" ("format string")) -> (spreadsheet string=w184:string)  [unwired: 1 in]
          n63 = Write to Text File(file (use dialog)=w186, text=w184, error in=w190) -> (refnum out=w185:refnum<file>, error out=w189:errorcluster)  [unwired: 1 in, 1 out]
          n64 = call "Get Error Byte.vi"("error"=w172) -> ("error  out"=w171:errorcluster, "Error Byte"=w170:u8)  [unwired: 9 in]
          n65 = Close File(refnum=w185, error in=w189) -> ()  [unwired: 2 out]
          n66 = call "Convert Boolean to DBL Array.vi"("Error Code"=w170, "Boolean"=w195) -> ("DBL Array"=w196:dbl[])  [unwired: 9 in]
          n67 = RT FIFO Write(0:w178, 1:w196) -> (11:w194:errorcluster)  [unwired: 3 in, 3 out]
          n68 = Merge Errors(w171, w194) -> (w193:errorcluster)
          n69 = call <vilib>:"Diag Set Property.vi"("error in (no error)"=w193, "property value"=w197, "property ID"=Property_ID."Timeout Diag Command", "diag ref in"=w174) -> ("error out"=w179:errorcluster, "diag ref out"=w173:T29)  [unwired: 6 in]
          n70 = in-place-cluster #6("Parameters.ChanRefs.ToVS.Status.Write to VS Engine FIFO"=w178, "ADCS Connection"=w173) -> (w164:T1)
        }
      }
      frame "UpdateDTCReport" {
        n71 = Unflatten From String(type=T33[] [] ("Active DTCs"), binary string=w204, error in (no error)=w208) -> (value=w210:T33[], error out=w207:errorcluster)  [unwired: 2 in, 1 out]
        n72 = Bundle By Name(cluster=w206, "Active DTCs"=w210) -> (w205:cluster{"Active DTCs":T33[], "status mask":u8})
      }
      frame "ConfigurePIDs" {
        n73 = in-place {
          in-place-border: w215 -> [w229]
          in-place-border: [w224] -> w214
          n74 = in-place-cluster #7(w213) -> ("Parameters.ChanRefs.ToVS.Status.Write to VS Engine FIFO"=w223:refnum<k33>, "Parameters.Properties.DPIDs"=w222:T15[], "ADCS Connection"=w221:T29)
          n75 = for {
            shift-right: [w236] -> w220
            shift-left: w221 -> [w237]
            tunnel: w222 -> [w235] mode=indexing
            shift-right: [w231] -> w219
            shift-left: w229 -> [w232]
            tunnel: [w230] -> w228 mode=indexing
            n76 = Unbundle By Name(w235) -> ("DPID ID"=w234:u8, "PIDs"=w233:u16[])
            n77 = call "GMLAN DynamicallyDefineMessage.vi"("error in (no error)"=w232, "PID List"=w233, "DPID ID"=w234, "diag ref in"=w237) -> ("error out"=w231:errorcluster, "success?"=w230:bool, "diag ref out"=w236:T29)  [unwired: 5 in]
          }
          n78 = And Array Elements(Boolean array=w228) -> (logical AND=w227:bool)
          n79 = call "Get Error Byte.vi"("error"=w219) -> ("error  out"=w218:errorcluster, "Error Byte"=w217:u8)  [unwired: 9 in]
          n80 = call "Convert Boolean to DBL Array.vi"("Error Code"=w217, "Boolean"=w227) -> ("DBL Array"=w226:dbl[])  [unwired: 9 in]
          n81 = RT FIFO Write(0:w223, 1:w226) -> (11:w225:errorcluster)  [unwired: 3 in, 3 out]
          n82 = in-place-cluster #7("Parameters.ChanRefs.ToVS.Status.Write to VS Engine FIFO"=w223, "Parameters.Properties.DPIDs"=w222, "ADCS Connection"=w220) -> (w212:T1)
          n83 = Merge Errors(w218, w225) -> (w224:errorcluster)
        }
      }
      frame "StartPIDs" {
        n84 = in-place {
          in-place-border: w239 -> [w261]
          in-place-border: [w259] -> w238
          w263 = Property_ID."Timeout Diag Command" ("property ID")
          w267 = T39[] [enum."scheduleAtSlowRate", enum."scheduleAtMediumRate", enum."scheduleAtFastRate"] items=["stopSending", "sendOneResponse", "scheduleAtSlowRate", "scheduleAtMediumRate", "scheduleAtFastRate"]
          n85 = in-place-cluster #8(w241) -> ("Parameters.ChanRefs.ToVS.Status.Write to VS Engine FIFO"=w251:refnum<k33>, "ADCS Connection"=w249:T29, "Parameters.Properties.DPIDs"=w252:T15[])
          n86 = call <vilib>:"Diag Get Property.vi"("error in (no error)"=w261, "property ID"=w263, "diag ref in"=w249) -> ("error out"=w265:errorcluster, "property value"=w258:u32, "diag ref out"=w250:T29)  [unwired: 6 in]
          n87 = call <vilib>:"Diag Set Property.vi"("error in (no error)"=w265, "property value"=u32 100, "property ID"=w263, "diag ref in"=w250) -> ("error out"=w260:errorcluster, "diag ref out"=w248:T29)  [unwired: 6 in]
          n88 = call "Sort DPID IDs by Speed.vi"("DPIDs"=w252) -> ("Filtered DPIDs IDs"=w266:T49)  [unwired: 10 in]
          n89 = for {
            tunnel: w266 -> [w273]
            shift-right: [w268] -> w245
            shift-left: w260 -> [w276]
            shift-right: [w274] -> w247
            shift-left: w248 -> [w275]
            tunnel: w267 -> [w270] mode=indexing
            tunnel: [w269] -> w255 mode=indexing
            stop <- w268 stop-if-true
            n90 = case shown="\"scheduleAtSlowRate\"" w270 {
              tunnel: w273 -> [w288 w290 _ w292]
              tunnel: [w287 w289 _ w291] -> w272
              frame "scheduleAtMediumRate" {
                n91 = Unbundle By Name(w288) -> ("Medium"=w287:u8[])
              }
              frame "scheduleAtFastRate" {
                n92 = Unbundle By Name(w290) -> ("Fast"=w289:u8[])
              }
              frame Default {
              }
              frame "scheduleAtSlowRate" {
                n93 = Unbundle By Name(w292) -> ("Slow"=w291:u8[])
              }
            }
            n94 = Empty Array?(array=w272) -> (empty?=w271:bool)
            n95 = case shown="False" w271 {
              tunnel: w276 -> [w283 w285]
              tunnel: [w282 w285] -> w268
              tunnel: w275 -> [w281 w286]
              tunnel: [w280 w286] -> w274
              tunnel: w270 -> [w277 _]
              tunnel: w272 -> [w279 _]
              tunnel: [w278 TRUE ("success?")] -> w269
              frame False {
                n96 = call "GMLAN ReadDataByPacketIdentifier.vi"("error in (no error)"=w283, "DPIDs"=w279, "Sub Function"=w277, "diag ref in"=w281) -> ("error out"=w282:errorcluster, "success?"=w278:bool, "diag ref out"=w280:T29)  [unwired: 4 in, 1 out]
              }
              frame True {
              }
            }
          }
          n97 = And Array Elements(Boolean array=w255) -> (logical AND=w257:bool)
          n98 = call "Get Error Byte.vi"("error"=w245) -> ("error  out"=w244:errorcluster, "Error Byte"=w243:u8)  [unwired: 9 in]
          n99 = call "Convert Boolean to DBL Array.vi"("Error Code"=w243, "Boolean"=w257) -> ("DBL Array"=w256:dbl[])  [unwired: 9 in]
          n100 = RT FIFO Write(0:w251, 1:w256) -> (11:w254:errorcluster)  [unwired: 3 in, 3 out]
          n101 = Merge Errors(w244, w254) -> (w253:errorcluster)
          n102 = call <vilib>:"Diag Set Property.vi"("error in (no error)"=w253, "property value"=w258, "property ID"=Property_ID."Timeout Diag Command", "diag ref in"=w247) -> ("error out"=w259:errorcluster, "diag ref out"=w246:T29)  [unwired: 6 in]
          n103 = in-place-cluster #8("Parameters.ChanRefs.ToVS.Status.Write to VS Engine FIFO"=w251, "ADCS Connection"=w246, "Parameters.Properties.DPIDs"=w252) -> (w240:T1)
        }
      }
      frame "StopPIDs" {
        n104 = in-place {
          in-place-border: w296 -> [w318]
          in-place-border: [w316] -> w295
          w320 = Property_ID."Timeout Diag Command" ("property ID")
          n105 = in-place-cluster #9(w294) -> ("Parameters.ChanRefs.ToVS.Status.Write to VS Engine FIFO"=w307:refnum<k33>, "ADCS Connection"=w304:T29, "Parameters.Properties.DPIDs"=w306:T15[])
          n106 = for {
            tunnel: w306 -> [w334] mode=indexing
            tunnel: [w333] -> w313 mode=indexing
            n107 = Unbundle By Name(w334) -> ("DPID ID"=w333:u8)
          }
          n108 = call <vilib>:"Diag Get Property.vi"("error in (no error)"=w318, "property ID"=w320, "diag ref in"=w304) -> ("error out"=w322:errorcluster, "property value"=w315:u32, "diag ref out"=w305:T29)  [unwired: 6 in]
          n109 = call <vilib>:"Diag Set Property.vi"("error in (no error)"=w322, "property value"=u32 100, "property ID"=w320, "diag ref in"=w305) -> ("error out"=w317:errorcluster, "diag ref out"=w303:T29)  [unwired: 6 in]
          n110 = Empty Array?(array=w313) -> (empty?=w314:bool)
          n111 = case shown="False" w314 {
            tunnel: w317 -> [w329 w331]
            tunnel: [w328 w331] -> w300
            tunnel: w303 -> [w327 w332]
            tunnel: [w326 w332] -> w302
            tunnel: ReadDataByPacketIdentifier_SubFunctions."stopSending" ("Sub Function") -> [w325 _]
            tunnel: w313 -> [w324 _]
            tunnel: [w323 TRUE ("success?")] -> w311
            frame False {
              n112 = call "GMLAN ReadDataByPacketIdentifier.vi"("error in (no error)"=w329, "DPIDs"=w324, "Sub Function"=w325, "diag ref in"=w327) -> ("error out"=w328:errorcluster, "success?"=w323:bool, "diag ref out"=w326:T29)  [unwired: 4 in, 1 out]
            }
            frame True {
            }
          }
          n113 = call "Get Error Byte.vi"("error"=w300) -> ("error  out"=w299:errorcluster, "Error Byte"=w298:u8)  [unwired: 9 in]
          n114 = call "Convert Boolean to DBL Array.vi"("Error Code"=w298, "Boolean"=w311) -> ("DBL Array"=w312:dbl[])  [unwired: 9 in]
          n115 = RT FIFO Write(0:w307, 1:w312) -> (11:w310:errorcluster)  [unwired: 3 in, 3 out]
          n116 = Merge Errors(w299, w310) -> (w309:errorcluster)
          n117 = call <vilib>:"Diag Set Property.vi"("error in (no error)"=w309, "property value"=w315, "property ID"=Property_ID."Timeout Diag Command", "diag ref in"=w302) -> ("error out"=w316:errorcluster, "diag ref out"=w301:T29)  [unwired: 6 in]
          n118 = in-place-cluster #9("Parameters.ChanRefs.ToVS.Status.Write to VS Engine FIFO"=w307, "ADCS Connection"=w301, "Parameters.Properties.DPIDs"=w306) -> (w293:T1)
        }
      }
      frame "<--------------- GENERIC SERVICES --------------->" {
      }
      frame "ForceTesterPresent" {
        # "#TODO Force a TesterPresent and Reset tester present timer."
      }
      frame "ClearSuccessBit" {
        n119 = in-place {
          in-place-border: w344 -> [w350]
          in-place-border: [w349] -> w343
          n120 = in-place-cluster #10(w342) -> ("Parameters.ChanRefs.ToVS.Status.Write to VS Engine FIFO"=w348:refnum<k33>)
          n121 = call "Convert Boolean to DBL Array.vi"("Error Code"=0.0, "Boolean"=FALSE) -> ("DBL Array"=w353:dbl[])  [unwired: 9 in]
          n122 = RT FIFO Write(0:w348, 1:w353) -> (8:w347:refnum<k33>, 11:w352:errorcluster)  [unwired: 3 in, 2 out]
          n123 = in-place-cluster #10("Parameters.ChanRefs.ToVS.Status.Write to VS Engine FIFO"=w347) -> (w341:T1)
          n124 = Merge Errors(w350, w352) -> (w349:errorcluster)
        }
      }
      frame "EnableDiagnosticSession" {
        n125 = in-place {
          in-place-border: w358 -> [w370]
          in-place-border: [w369] -> w357
          in-place-border: w356 -> [w368]
          n126 = in-place-cluster #11(w355) -> ("Parameters.ChanRefs.ToVS.Status.Write to VS Engine FIFO"=w365:refnum<k33>, "Parameters.Properties.CAN.Diagnostic Protocol"=w363:T9, "ADCS Connection"=w367:T29)
          n127 = Unflatten From String(type=u8 0 ("ID"), binary string=w368, error in (no error)=w370) -> (value=w372:u8, error out=w371:errorcluster)  [unwired: 2 in, 1 out]
          n128 = case shown="\"UDS\"" w363 {
            tunnel: [w380 w389 w392] -> w362
            tunnel: [w382 w388 w391] -> w374
            tunnel: w372 -> [w377 w387 w394]
            tunnel: w371 -> [w381 w386 w393]
            tunnel: w367 -> [w379 w385 w395]
            tunnel: [w378 w384 w390] -> w366
            frame "GMLAN" {
              n129 = call "GMLAN InitiateDiagnosticOperation.vi"("error in (no error)"=w381, "SubFunctions"=w377, "Parameter"=InitiateDiagnosticOperation_Parameter."SpecificECU", "diag ref in"=w379) -> ("error out"=w380:errorcluster, "success?"=w382:bool, "diag ref out"=w378:T29)  [unwired: 5 in]
            }
            frame "UDS" {
              n130 = call <vilib>:"UDS DiagnosticSessionControl.vi"("error in (no error)"=w386, "mode"=w387, "diag ref in"=w385) -> ("error out"=w389:errorcluster, "success?"=w388:bool, "diag ref out"=w384:T29)  [unwired: 5 in, 1 out]
            }
            frame "KWP-2000" {
              n131 = call <vilib>:"StartDiagnosticSession.vi"("error in (no error)"=w393, "mode"=w394, "diag ref in"=w395) -> ("error out"=w392:errorcluster, "success?"=w391:bool, "diag ref out"=w390:T29)  [unwired: 6 in]
            }
          }
          n132 = call "Get Error Byte.vi"("error"=w362) -> ("error  out"=w361:errorcluster, "Error Byte"=w360:u8)  [unwired: 9 in]
          n133 = call "Convert Boolean to DBL Array.vi"("Error Code"=w360, "Boolean"=w374) -> ("DBL Array"=w376:dbl[])  [unwired: 9 in]
          n134 = RT FIFO Write(0:w365, 1:w376) -> (8:w364:refnum<k33>, 11:w375:errorcluster)  [unwired: 3 in, 2 out]
          n135 = in-place-cluster #11("Parameters.ChanRefs.ToVS.Status.Write to VS Engine FIFO"=w364, "Parameters.Properties.CAN.Diagnostic Protocol"=w363, "ADCS Connection"=w366) -> (w354:T1)
          n136 = Merge Errors(w361, w375) -> (w369:errorcluster)
        }
      }
      frame "DisableDiagnosticSession" {
        n137 = in-place {
          in-place-border: [w410] -> w399
          in-place-border: w398 -> [w409]
          n138 = in-place-cluster #12(w397) -> ("Parameters.ChanRefs.ToVS.Status.Write to VS Engine FIFO"=w406:refnum<k33>, "Parameters.Properties.CAN.Diagnostic Protocol"=w404:T9, "ADCS Connection"=w408:T29)
          n139 = case shown="\"GMLAN\"" w404 {
            tunnel: [w416 w422 w431] -> w403
            tunnel: [w418 w421 w430] -> w411
            tunnel: w409 -> [w415 w425 w428]
            tunnel: w408 -> [w414 w424 w427]
            tunnel: [w417 w423 w426] -> w407
            frame "GMLAN" {
              w419 = T50 2 items=["disableAllDTCs"=2, "enableDTCsDuringDevCntrl"=3, "wakeUpLinks"=4] ("SubFunctions")
              n140 = call "GMLAN InitiateDiagnosticOperation.vi"("error in (no error)"=w415, "SubFunctions"=w419, "Parameter"=InitiateDiagnosticOperation_Parameter."SpecificECU", "diag ref in"=w414) -> ("error out"=w416:errorcluster, "success?"=w418:bool, "diag ref out"=w417:T29)  [unwired: 5 in]
            }
            frame "KWP-2000" {
              n141 = call <vilib>:"StopDiagnosticSession.vi"("error in (no error)"=w425, "diag ref in"=w424) -> ("error out"=w422:errorcluster, "success?"=w421:bool, "diag ref out"=w423:T29)  [unwired: 7 in]
            }
            frame "UDS" {
              n142 = call <vilib>:"UDS DiagnosticSessionControl.vi"("error in (no error)"=w428, "mode"=u8 1, "diag ref in"=w427) -> ("error out"=w431:errorcluster, "success?"=w430:bool, "diag ref out"=w426:T29)  [unwired: 5 in, 1 out]
            }
          }
          n143 = call "Get Error Byte.vi"("error"=w403) -> ("error  out"=w402:errorcluster, "Error Byte"=w401:u8)  [unwired: 9 in]
          n144 = call "Convert Boolean to DBL Array.vi"("Error Code"=w401, "Boolean"=w411) -> ("DBL Array"=w413:dbl[])  [unwired: 9 in]
          n145 = RT FIFO Write(0:w406, 1:w413) -> (8:w405:refnum<k33>, 11:w412:errorcluster)  [unwired: 3 in, 2 out]
          n146 = in-place-cluster #12("Parameters.ChanRefs.ToVS.Status.Write to VS Engine FIFO"=w405, "Parameters.Properties.CAN.Diagnostic Protocol"=w404, "ADCS Connection"=w407) -> (w396:T1)
          n147 = Merge Errors(w402, w412) -> (w410:errorcluster)
        }
      }
      frame "DisableNormalCommunication" {
        n148 = in-place {
          in-place-border: [w447] -> w435
          in-place-border: w434 -> [w445]
          n149 = in-place-cluster #13(w433) -> ("Parameters.ChanRefs.ToVS.Status.Write to VS Engine FIFO"=w442:refnum<k33>, "Parameters.Properties.CAN.Diagnostic Protocol"=w440:T9, "ADCS Connection"=w444:T29)
          n150 = case shown="\"UDS\"" w440 {
            tunnel: w444 -> [w450 w462 w467]
            tunnel: [w451 w461 w466] -> w443
            tunnel: [w453 w460 w464] -> w439
            tunnel: [w452 w459 w465] -> w446
            tunnel: w445 -> [w454 w456 w468]
            frame "GMLAN" {
              n151 = call "GMLAN DisableNormalCommunication.vi"("error in (no error)"=w454, "Parameter"=DisableNormalCommunication_Parameter."SpecificECU", "diag ref in"=w450) -> ("error out"=w453:errorcluster, "success?"=w452:bool, "diag ref out"=w451:T29)  [unwired: 6 in]
            }
            frame "UDS" {
              n152 = call <vilib>:"UDS CommunicationControl.vi"("error in (no error)"=w456, "communication type"=u8 3, "type"=u8 3, "diag ref in"=w462) -> ("error out"=w460:errorcluster, "success?"=w459:bool, "diag ref out"=w461:T29)  [unwired: 5 in]
            }
            frame "KWP-2000" {
              n153 = call <vilib>:"DisableNormalMessageTransmission.vi"("error in (no error)"=w468, "require response?"=TRUE, "diag ref in"=w467) -> ("error out"=w464:errorcluster, "success?"=w465:bool, "diag ref out"=w466:T29)  [unwired: 6 in]
            }
          }
          n154 = call "Get Error Byte.vi"("error"=w439) -> ("error  out"=w438:errorcluster, "Error Byte"=w437:u8)  [unwired: 9 in]
          n155 = call "Convert Boolean to DBL Array.vi"("Error Code"=w437, "Boolean"=w446) -> ("DBL Array"=w449:dbl[])  [unwired: 9 in]
          n156 = RT FIFO Write(0:w442, 1:w449) -> (8:w441:refnum<k33>, 11:w448:errorcluster)  [unwired: 3 in, 2 out]
          n157 = Merge Errors(w438, w448) -> (w447:errorcluster)
          n158 = in-place-cluster #13("Parameters.ChanRefs.ToVS.Status.Write to VS Engine FIFO"=w441, "Parameters.Properties.CAN.Diagnostic Protocol"=w440, "ADCS Connection"=w443) -> (w432:T1)
        }
      }
      frame "ReturnToNormalMode" {
        n159 = in-place {
          in-place-border: [w484] -> w472
          in-place-border: w471 -> [w482]
          n160 = in-place-cluster #14(w470) -> ("Parameters.ChanRefs.ToVS.Status.Write to VS Engine FIFO"=w479:refnum<k33>, "ADCS Connection"=w481:T29, "Parameters.Properties.CAN.Diagnostic Protocol"=w477:T9)
          n161 = case shown="\"UDS\"" w477 {
            tunnel: [w489 w498 w500] -> w476
            tunnel: [w487 w497 w501] -> w483
            tunnel: w482 -> [w491 w494 w504]
            tunnel: w481 -> [w490 w493 w503]
            tunnel: [w488 w492 w502] -> w480
            frame "GMLAN", Default {
              n162 = call "GMLAN ReturnToNormalMode.vi"("error in (no error)"=w491, "diag ref in"=w490) -> ("error out"=w489:errorcluster, "success?"=w487:bool, "diag ref out"=w488:T29)  [unwired: 7 in]
            }
            frame "UDS" {
              n163 = call <vilib>:"UDS CommunicationControl.vi"("error in (no error)"=w494, "communication type"=u8 3 ("type"), "type"=u8 0, "diag ref in"=w493) -> ("error out"=w498:errorcluster, "success?"=w497:bool, "diag ref out"=w492:T29)  [unwired: 5 in]
            }
            frame "KWP-2000" {
              n164 = call <vilib>:"EnableNormalMessageTransmission.vi"("error in (no error)"=w504, "require response?"=TRUE, "diag ref in"=w503) -> ("error out"=w500:errorcluster, "success?"=w501:bool, "diag ref out"=w502:T29)  [unwired: 6 in]
            }
          }
          n165 = call "Get Error Byte.vi"("error"=w476) -> ("error  out"=w475:errorcluster, "Error Byte"=w474:u8)  [unwired: 9 in]
          n166 = call "Convert Boolean to DBL Array.vi"("Error Code"=w474, "Boolean"=w483) -> ("DBL Array"=w486:dbl[])  [unwired: 9 in]
          n167 = RT FIFO Write(0:w479, 1:w486) -> (8:w478:refnum<k33>, 11:w485:errorcluster)  [unwired: 3 in, 2 out]
          n168 = Merge Errors(w475, w485) -> (w484:errorcluster)
          n169 = in-place-cluster #14("Parameters.ChanRefs.ToVS.Status.Write to VS Engine FIFO"=w478, "ADCS Connection"=w480, "Parameters.Properties.CAN.Diagnostic Protocol"=w477) -> (w469:T1)
        }
      }
      frame "UnlockECU" {
        n170 = in-place {
          in-place-border: w508 -> [w523]
          in-place-border: [w519] -> w507
          n171 = in-place-cluster #15(w506) -> ("Parameters.ChanRefs.ToVS.Status.Write to VS Engine FIFO"=w516:refnum<k33>, "ADCS Connection"=w518:T29, "Parameters.Properties.CAN.Security"=w517:T11, "Parameters.Properties.CAN.Diagnostic Protocol"=w513:T9)
          n172 = call "Unlock ECU Security.vi"("Diagnostic Protocol"=w513, "error in (no error)"=w523, "Security"=w517, "diag ref in"=w518) -> ("error out"=w512:errorcluster, "success?"=w520:bool, "diag ref out"=w514:T29)  [unwired: 5 in]
          n173 = call "Get Error Byte.vi"("error"=w512) -> ("error  out"=w511:errorcluster, "Error Byte"=w510:u8)  [unwired: 9 in]
          n174 = call "Convert Boolean to DBL Array.vi"("Error Code"=w510, "Boolean"=w520) -> ("DBL Array"=w522:dbl[])  [unwired: 9 in]
          n175 = RT FIFO Write(0:w516, 1:w522) -> (8:w515:refnum<k33>, 11:w521:errorcluster)  [unwired: 3 in, 2 out]
          n176 = Merge Errors(w511, w521) -> (w519:errorcluster)
          n177 = in-place-cluster #15("Parameters.ChanRefs.ToVS.Status.Write to VS Engine FIFO"=w515, "ADCS Connection"=w514, "Parameters.Properties.CAN.Security"=w517, "Parameters.Properties.CAN.Diagnostic Protocol"=w513) -> (w505:T1)
        }
      }
      frame "ReadActiveDTCs" {
        n178 = in-place {
          in-place-border: [w553] -> w532
          in-place-border: w531 -> [w552]
          in-place-border: w530 -> [w551]
          in-place-border: w529 -> [w550]
          in-place-border: w528 -> [w549]
          n179 = in-place-cluster #16(w527) -> ("Parameters.ChanRefs.ToVS.Status.Write to VS Engine FIFO"=w544:refnum<k33>, "Parameters.ChanRefs.ToVS.DTCCount.Write to VS Engine FIFO"=w540:refnum<k33>, "Parameters.ChanRefs.ToVS.DTCs.Write to VS Engine FIFO"=w539:refnum<k33>, "Parameters.ChanRefs.ToVS.DTCs.Pairs.Values"=w547:dbl[], "Parameters.Properties.DTC descriptor"=w542:T17, "ADCS Connection"=w546:T29, "Parameters.Properties.CAN.Diagnostic Protocol"=w538:T9)
          n180 = in-place-cluster #17(w526) -> ("Active DTCs"=w548:T33[])
          n181 = case shown="Default" w538 {
            selector: w538 -> [w570 w577]
            tunnel: [w562 w601] -> w553
            tunnel: w552 -> [w561 w600]
            tunnel: w551 -> [w563 w594]
            tunnel: w550 -> [_ w593]
            tunnel: w549 -> [_ w592]
            tunnel: w548 -> [w560 w584]
            tunnel: w547 -> [w557 w583]
            tunnel: w546 -> [w559 w582]
            tunnel: [w560 w581] -> w545
            tunnel: w544 -> [w554 w574]
            tunnel: [w557 w580] -> w543
            tunnel: w542 -> [w558 w573]
            tunnel: [w559 w579] -> w541
            tunnel: w540 -> [w555 w575]
            tunnel: w539 -> [w556 w576]
            tunnel: [w570 w577] -> w537
            tunnel: [w558 w573] -> w536
            tunnel: [w556 w576] -> w535
            tunnel: [w555 w575] -> w534
            tunnel: [w554 w574] -> w533
            frame "GMLAN" {
              n182 = global read "GUID Lookup.vi" "ResponseQKey"() -> (w565:string)
              n183 = Unbundle By Name(w561) -> ("attributes"=w564:T47)
              n184 = Flatten To String(anything=w560, error in (no error)=w563) -> (data string=w567:string, error out=w568:errorcluster)  [unwired: 2 in, 1 out]
              n185 = call <vilib>:"Index.vi"("key"=w565, "array in"=w564) -> ("value"=w566:string)  [unwired: 3 in, 2 out]
              n186 = call <vilib>:"Send Local Message.vi"("receiver process (\"\" - local)"=w566, "message name"="ActiveDTCs" ("Message Name"), "message value"=w567, "error in"=w568) -> ("error out"=w562:errorcluster)  [unwired: 9 in, 2 out]
            }
            frame Default {
              n187 = Unflatten From String(type=u32[] [], binary string=w593, error in (no error)=w594) -> (value=w588:u32[], error out=w590:errorcluster)  [unwired: 2 in, 1 out]
              n188 = case shown="\"KWP-2000\"" w577 {
                tunnel: w573 -> [w612 w646 _]
                tunnel: w590 -> [w605 w641 w666]
                tunnel: w582 -> [w604 w640 w667]
                tunnel: [w606 w642 _] -> w589
                tunnel: w588 -> [w611 w648 _]
                tunnel: [w609 w643 w666] -> w572
                tunnel: [w608 w645 w667] -> w579
                tunnel: [w607 w644 _] -> w585
                frame "UDS" {
                  n189 = Index Array(array=w611) -> (element #1=w603:u32, element #2=w610:u32, element #3=w602:u32)  [unwired: 3 in]
                  n190 = case shown="1" w603 {
                    tunnel: w612 -> [w616 w623 w637]
                    tunnel: w610 -> [w614 w622 w636]
                    tunnel: [w620 w628 w635] -> w609
                    tunnel: [w617 w625 w634] -> w608
                    tunnel: [w618 w626 w633] -> w607
                    tunnel: [w619 w627 w632] -> w606
                    tunnel: w605 -> [w621 w629 w631]
                    tunnel: w604 -> [w615 w624 w630]
                    tunnel: w602 -> [w613 _ _]
                    frame 1 {
                      n191 = call <vilib>:"UDS ReportDTCBySeverityMaskRecord.vi"("DTC descriptor"=w616, "error in (no error)"=w621, "status"=w614, "severity mask"=w613, "diag ref in"=w615) -> ("error out"=w620:errorcluster, "success?"=w619:bool, "DTCs"=w618:T51[], "diag ref out"=w617:T29)  [unwired: 2 in, 1 out]
                    }
                    frame 2 {
                      n192 = call <vilib>:"UDS ReportSeverityInformationOfDTC.vi"("DTC descriptor"=w623, "error in (no error)"=w629, "DTC mask record"=w622, "diag ref in"=w624) -> ("error out"=w628:errorcluster, "success?"=w627:bool, "DTCs"=w626:T51[], "diag ref out"=w625:T29)  [unwired: 3 in, 1 out]
                    }
                    frame 0, Default {
                      n193 = call <vilib>:"UDS ReportDTCByStatusMask.vi"("DTC descriptor"=w637, "error in (no error)"=w631, "status mask"=w636, "diag ref in"=w630) -> ("error out"=w635:errorcluster, "success?"=w632:bool, "DTCs"=w633:T51[], "diag ref out"=w634:T29)  [unwired: 3 in, 1 out]
                    }
                  }
                }
                frame "KWP-2000" {
                  n194 = Index Array(array=w648) -> (element #1=w639:u32, element #2=w647:u32, element #3=w638:u32)  [unwired: 3 in]
                  n195 = case shown="1" w639 {
                    tunnel: w647 -> [w656 w665]
                    tunnel: w646 -> [w655 w664]
                    tunnel: [w654 w663] -> w645
                    tunnel: [w653 w662] -> w644
                    tunnel: [w652 w661] -> w643
                    tunnel: [w651 w660] -> w642
                    tunnel: w641 -> [w650 w659]
                    tunnel: w640 -> [w649 w658]
                    tunnel: w638 -> [_ w657]
                    frame 0, Default {
                      n196 = call <vilib>:"ReadStatusOfDTC.vi"("DTC descriptor"=w655, "error in (no error)"=w650, "group of DTC"=w656, "diag ref in"=w649) -> ("error out"=w652:errorcluster, "success?"=w651:bool, "DTCs"=w653:T51[], "diag ref out"=w654:T29)  [unwired: 4 in]
                    }
                    frame 1 {
                      n197 = call <vilib>:"ReadDTCByStatus.vi"("DTC descriptor"=w664, "error in (no error)"=w659, "group of DTC"=w665, "mode"=w657, "diag ref in"=w658) -> ("error out"=w661:errorcluster, "success?"=w660:bool, "DTCs"=w662:T51[], "diag ref out"=w663:T29)  [unwired: 3 in]
                    }
                  }
                }
                frame "GMLAN" {
                }
              }
              n198 = case shown="No Error" w572 {
                selector: w572 -> [w683 w707]
                tunnel: w576 -> [w686 _]
                tunnel: w592 -> [w694 _]
                tunnel: w583 -> [w693 w708]
                tunnel: [w692 w708] -> w580
                tunnel: [w684 w707] -> w591
                tunnel: w575 -> [w687 _]
                tunnel: w585 -> [w690 _]
                tunnel: w584 -> [w689 w706]
                tunnel: [w688 w706] -> w581
                frame No Error {
                  n199 = Get Date/Time In Seconds() -> (seconds since 1Jan1904=w682:timestamp)
                  n200 = call "Determine Active DTCs and Timestamps.vi"("current time"=w682, "Previous Changed DTCs"=w689, "current DTCs"=w690) -> ("Active DTCs"=w688:T33[])  [unwired: 8 in]
                  n201 = Replace Array Subset(array=w694, new element=w688, index=0) -> (w696:T33[])
                  n202 = for {
                    tunnel: w696 -> [w705] mode=indexing
                    shift-right: [w704] -> w692
                    shift-left: w693 -> [w703]
                    i -> [w700]
                    # "Put 10 newest DTCs in VS"
                    n203 = Cluster To Array(cluster=w705) -> (array=w702:dbl[])
                    n204 = Array Size(array=w702) -> (size(s)=w701:i32)
                    n205 = Multiply(x=w701, y=w700) -> (x*y=w699:i32)
                    n206 = Replace Array Subset(array=w703, new element=w702, index=w699) -> (w704:dbl[])
                  }
                  n207 = Array Size(array=w688) -> (size(s)=w697:i32)
                  n208 = To Double Precision Float(number=w697) -> (double precision float=w698:dbl)
                  n209 = Build Array(w698) -> (w691:dbl[])
                  n210 = RT FIFO Write(0:w687, 1:w691, 3:w683) -> (11:w685:errorcluster)  [unwired: 2 in, 3 out]
                  n211 = RT FIFO Write(0:w686, 1:w692, 3:w685) -> (11:w684:errorcluster)  [unwired: 2 in, 3 out]
                }
                frame Error {
                }
              }
              n212 = call "Get Error Byte.vi"("error"=w572) -> ("Error Byte"=w571:u8)  [unwired: 9 in, 1 out]
              n213 = global read "GUID Lookup.vi" "ResponseQKey"() -> (w599:string)
              n214 = Unbundle By Name(w600) -> ("attributes"=w586:T47)
              n215 = call "Convert Boolean to DBL Array.vi"("Error Code"=w571, "Boolean"=w589) -> ("DBL Array"=w596:dbl[])  [unwired: 9 in]
              n216 = call <vilib>:"Index.vi"("key"=w599, "array in"=w586) -> ("value"=w597:string)  [unwired: 3 in, 2 out]
              n217 = RT FIFO Write(0:w574, 1:w596) -> (11:w595:errorcluster)  [unwired: 3 in, 3 out]
              n218 = Empty String/Path?(string/path=w597) -> (empty?=w598:bool)
              n219 = Merge Errors(w591, w595) -> (w587:errorcluster)
              n220 = case shown="No Error" w587 {
                selector: w587 -> [w669 w681]
                tunnel: [w672 w681] -> w601
                tunnel: w598 -> [w671 _]
                tunnel: w597 -> [w670 _]
                tunnel: w581 -> [w668 _]
                frame No Error {
                  n221 = case shown="False" w671 {
                    tunnel: [w679 w680] -> w672
                    tunnel: w669 -> [w675 w680]
                    tunnel: w670 -> [w674 _]
                    tunnel: w668 -> [w673 _]
                    frame False {
                      # "send ALL DTCs to TCP engine"
                      n222 = Flatten To String(anything=w673, error in (no error)=w675) -> (data string=w676:string, error out=w677:errorcluster)  [unwired: 2 in, 1 out]
                      n223 = call <vilib>:"Send Local Message.vi"("receiver process (\"\" - local)"=w674, "message name"="ActiveDTCs" ("Message Name"), "message value"=w676, "error in"=w677) -> ("error out"=w679:errorcluster)  [unwired: 9 in, 2 out]
                    }
                    frame True {
                    }
                  }
                }
                frame Error {
                }
              }
            }
          }
          n224 = in-place-cluster #16("Parameters.ChanRefs.ToVS.Status.Write to VS Engine FIFO"=w533, "Parameters.ChanRefs.ToVS.DTCCount.Write to VS Engine FIFO"=w534, "Parameters.ChanRefs.ToVS.DTCs.Write to VS Engine FIFO"=w535, "Parameters.ChanRefs.ToVS.DTCs.Pairs.Values"=w543, "Parameters.Properties.DTC descriptor"=w536, "ADCS Connection"=w541, "Parameters.Properties.CAN.Diagnostic Protocol"=w537) -> (w524:T1)
          n225 = in-place-cluster #17("Active DTCs"=w545) -> (w525:cluster{"Active DTCs":T33[], "status mask":u8})
        }
      }
      frame "ControlDTC" {
        n226 = in-place {
          in-place-border: w711 -> [w731]
          in-place-border: [w726] -> w710
          in-place-border: w709 -> [w730]
          n227 = in-place-cluster #18(w713) -> ("Parameters.ChanRefs.ToVS.Status.Write to VS Engine FIFO"=w733:refnum<k33>, "Parameters.Properties.DTC descriptor"=w738:T17, "ADCS Connection"=w737:T29, "Parameters.Properties.CAN.Diagnostic Protocol"=w739:T9, "Parameters.ChanRefs.FromVS.DTCControl.Read from VS Engine FIFO"=w717:refnum<k33>, "Parameters.ChanRefs.FromVS.DTCControl.Pairs.Values"=w715:dbl[])
          n228 = Unflatten From String(type=u32 0, binary string=w730, error in (no error)=w731) -> (value=w728:u32, error out=w724:errorcluster)  [unwired: 2 in, 1 out]
          n229 = RT FIFO Read(0:w717, 1:w715, 3:w724) -> (8:w716:refnum<k33>, 9:w721:dbl[], 11:w720:errorcluster)  [unwired: 1 in, 2 out]
          n230 = call-poly <vilib>:"XNET Convert.vi"("signal data"=w721, "error in (no error)"=w720) -> ("frame data"=w723:u8[], "error out"=w719:errorcluster)  [unwired: 11 in, 1 out]
          n231 = Array Subset(array=w723, index=16) -> (w718:u8[])  [unwired: 1 in]
          n232 = case shown="\"KWP-2000\"" w739 {
            tunnel: w719 -> [w742 w748 w756]
            tunnel: [w742 w747 w755] -> w727
            tunnel: w738 -> [_ _ w754]
            tunnel: w737 -> [w741 w745 w753]
            tunnel: [w741 w746 w752] -> w736
            tunnel: [FALSE ("success?") w744 w751] -> w734
            tunnel: w728 -> [_ w743 w750]
            tunnel: w718 -> [_ _ w749]
            frame "GMLAN", Default {
            }
            frame "UDS" {
              n233 = call <vilib>:"UDS ControlDTCSetting.vi"("error in (no error)"=w748, "type"=w743, "diag ref in"=w745) -> ("error out"=w747:errorcluster, "success?"=w744:bool, "diag ref out"=w746:T29)  [unwired: 6 in]
            }
            frame "KWP-2000" {
              n234 = call <vilib>:"ControlDTCSetting.vi"("DTC descriptor"=w754, "error in (no error)"=w756, "group of DTC"=w750, "data in"=w749, "diag ref in"=w753) -> ("error out"=w755:errorcluster, "success?"=w751:bool, "diag ref out"=w752:T29)  [unwired: 4 in]
            }
          }
          n235 = call "Get Error Byte.vi"("error"=w727) -> ("error  out"=w726:errorcluster, "Error Byte"=w725:u8)  [unwired: 9 in]
          n236 = call "Convert Boolean to DBL Array.vi"("Error Code"=w725, "Boolean"=w734) -> ("DBL Array"=w735:dbl[])  [unwired: 9 in]
          n237 = RT FIFO Write(0:w733, 1:w735) -> (8:w732:refnum<k33>)  [unwired: 3 in, 3 out]
          n238 = in-place-cluster #18("Parameters.ChanRefs.ToVS.Status.Write to VS Engine FIFO"=w732, "Parameters.Properties.DTC descriptor"=w738, "ADCS Connection"=w736, "Parameters.Properties.CAN.Diagnostic Protocol"=w739, "Parameters.ChanRefs.FromVS.DTCControl.Read from VS Engine FIFO"=w716) -> (w712:T1)  [unwired: 1 in]
        }
      }
      frame "ClearDTCs" {
        n239 = in-place {
          in-place-border: w763 -> [w789]
          in-place-border: w762 -> [w788]
          in-place-border: [w784] -> w761
          in-place-border: w760 -> [w783]
          in-place-border: w759 -> [w782]
          n240 = in-place-cluster #19(w758) -> ("Parameters.ChanRefs.ToVS.Status.Write to VS Engine FIFO"=w767:refnum<k33>, "Parameters.ChanRefs.ToVS.DTCCount.Write to VS Engine FIFO"=w775:refnum<k33>, "Parameters.ChanRefs.ToVS.DTCs.Write to VS Engine FIFO"=w776:refnum<k33>, "Parameters.ChanRefs.ToVS.DTCs.Pairs.Values"=w778:dbl[], "Parameters.Properties.DTC descriptor"=w779:T17, "Parameters.Properties.CAN.Diagnostic Protocol"=w772:T9, "ADCS Connection"=w781:T29, "XNETEngine (GMLAN)"=w770:T32)
          n241 = case shown="Default" w772 {
            selector: w772 -> [w807 w817]
            tunnel: w789 -> [w790 w842]
            tunnel: w788 -> [w795 w840]
            tunnel: [w794 w839] -> w786
            tunnel: [w793 w831] -> w766
            tunnel: w783 -> [_ w828]
            tunnel: w782 -> [w803 w827]
            tunnel: w781 -> [w800 w824]
            tunnel: [w799 w823] -> w780
            tunnel: w779 -> [_ w822]
            tunnel: w778 -> [w798 w821]
            tunnel: [w798 w820] -> w777
            tunnel: w776 -> [w809 w818]
            tunnel: w775 -> [w808 w819]
            tunnel: [w808 w819] -> w774
            tunnel: [w809 w818] -> w773
            tunnel: [w807 w817] -> w771
            tunnel: w770 -> [w792 w816]
            tunnel: [w792 w816] -> w769
            tunnel: [w791 w815] -> w768
            tunnel: w767 -> [w791 w815]
            frame "GMLAN" {
              n242 = global read "GUID Lookup.vi" "ResponseQKey"() -> (w805:string)
              n243 = Unbundle By Name(w790) -> ("attributes"=w804:T47)
              n244 = call <vilib>:"Send Local Message.vi"("message queue in"=w792, "message name"="ClearDTCs" ("Message Name"), "error in"=w803) -> ("error out"=w801:errorcluster)  [unwired: 10 in, 2 out]
              n245 = call <vilib>:"Index.vi"("key"=w805, "array in"=w804) -> ("value"=w796:string)  [unwired: 3 in, 2 out]
              n246 = call "GMLAN ClearDiagnosticInformation.vi"("error in (no error)"=w801, "diag ref in"=w800) -> ("error out"=w802:errorcluster, "success?"=w794:bool, "diag ref out"=w799:T29)  [unwired: 7 in]
              n247 = Empty String/Path?(string/path=w796) -> (empty?=w806:bool)
              n248 = case shown="True" w806 {
                tunnel: w802 -> [w810 w814]
                tunnel: [w810 w814] -> w793
                tunnel: w796 -> [w812 _]
                tunnel: w795 -> [w811 _]
                frame False {
                  n249 = call <vilib>:"Send Local Message.vi"("receiver process (\"\" - local)"=w812, "message name"=w811, "message value"="Cleared" ("Message Value")) -> ()  [unwired: 10 in, 3 out]
                }
                frame True {
                }
              }
            }
            frame Default {
              (unwired) u32 16777215 items=["All"=16777215] ("Group of DTC")
              n250 = Unflatten From String(type=u32 0 ("ID"), binary string=w828, error in (no error)=w827) -> (value=w825:u32, error out=w826:errorcluster)  [unwired: 2 in, 1 out]
              n251 = global read "GUID Lookup.vi" "ResponseQKey"() -> (w841:string)
              n252 = Array Size(array=w821) -> (size(s)=w837:i32)
              n253 = Unbundle By Name(w842) -> ("attributes"=w830:T47)
              n254 = case shown="\"UDS\"" w817 {
                tunnel: w824 -> [w846 w851 w860]
                tunnel: [w846 w850 w859] -> w823
                tunnel: [w845 w848 w858] -> w843
                tunnel: [FALSE ("success?") w849 w857] -> w839
                tunnel: w822 -> [_ w847 w856]
                tunnel: w826 -> [w845 w853 w855]
                tunnel: w825 -> [_ w852 w854]
                frame "GMLAN" {
                }
                frame "KWP-2000" {
                  n255 = call <vilib>:"ClearDiagnosticInformation.vi"("DTC descriptor"=w847, "error in (no error)"=w853, "group of DTC"=w852, "diag ref in"=w851) -> ("error out"=w848:errorcluster, "success?"=w849:bool, "diag ref out"=w850:T29)  [unwired: 5 in]
                }
                frame "UDS" {
                  n256 = call <vilib>:"UDS ClearDiagnosticInformation.vi"("DTC descriptor"=w856, "error in (no error)"=w855, "group of DTC"=w854, "diag ref in"=w860) -> ("error out"=w858:errorcluster, "success?"=w857:bool, "diag ref out"=w859:T29)  [unwired: 5 in]
                }
              }
              n257 = Initialize Array(0.0 ("element"), w837) -> (w820:dbl[])
              n258 = call <vilib>:"Index.vi"("key"=w841, "array in"=w830) -> ("value"=w835:string)  [unwired: 3 in, 2 out]
              n259 = Empty String/Path?(string/path=w835) -> (empty?=w834:bool)
              n260 = case shown="False" w834 {
                tunnel: w843 -> [w861 w865]
                tunnel: [w861 w865] -> w838
                tunnel: w835 -> [w863 _]
                tunnel: w840 -> [w862 _]
                frame False {
                  n261 = call <vilib>:"Send Local Message.vi"("receiver process (\"\" - local)"=w863, "message name"=w862, "message value"="Cleared" ("Message Value")) -> ()  [unwired: 10 in, 3 out]
                }
                frame True {
                }
              }
              n262 = RT FIFO Write(0:w818, 1:w820, 3:w838) -> (11:w832:errorcluster)  [unwired: 2 in, 3 out]
              n263 = RT FIFO Write(0:w819, 1:dbl[] [0.0] ("element"), 3:w832) -> (11:w831:errorcluster)  [unwired: 2 in, 3 out]
            }
          }
          n264 = call "Get Error Byte.vi"("error"=w766) -> ("error  out"=w765:errorcluster, "Error Byte"=w764:u8)  [unwired: 9 in]
          n265 = call "Convert Boolean to DBL Array.vi"("Error Code"=w764, "Boolean"=w786) -> ("DBL Array"=w787:dbl[])  [unwired: 9 in]
          n266 = in-place-cluster #19("Parameters.ChanRefs.ToVS.Status.Write to VS Engine FIFO"=w768, "Parameters.ChanRefs.ToVS.DTCCount.Write to VS Engine FIFO"=w774, "Parameters.ChanRefs.ToVS.DTCs.Write to VS Engine FIFO"=w773, "Parameters.ChanRefs.ToVS.DTCs.Pairs.Values"=w777, "Parameters.Properties.DTC descriptor"=w779, "Parameters.Properties.CAN.Diagnostic Protocol"=w771, "ADCS Connection"=w780, "XNETEngine (GMLAN)"=w769) -> (w757:T1)
          n267 = RT FIFO Write(0:w768, 1:w787) -> (11:w785:errorcluster)  [unwired: 3 in, 3 out]
          n268 = Merge Errors(w765, w785) -> (w784:errorcluster)
        }
      }
      frame "GenerateCPID" {
        n269 = disable-structure shown="Enabled" {
          disable-tunnel: w870 -> [w876 w920]
          disable-tunnel: w869 -> [w875 w919]
          disable-tunnel: [w874 w918] -> w868
          disable-tunnel: w867 -> [w873 w917]
          disable-tunnel: [w872 w916] -> w866
          frame Disabled {
            n270 = in-place {
              in-place-border: w876 -> [w894]
              in-place-border: w875 -> [w893]
              in-place-border: [w884] -> w874
              (unwired) u16 0
              n271 = in-place-cluster #20(w873) -> ("Parameters.ChanRefs.ToVS.Status.Write to VS Engine FIFO"=w879:refnum<k33>, "ADCS Connection"=w881:T29, "Parameters.Properties.CAN.Diagnostic Protocol"=w877:T9)
              n272 = Unflatten From String(type=u8[] [], binary string=w893, error in (no error)=w894) -> (value=w891:u8[], error out=w882:errorcluster)  [unwired: 2 in, 1 out]
              n273 = Delete From Array(array=w891, index=0) -> (deleted portion=w889:u8, array with subset deleted=w888:u8[])  [unwired: 1 in]
              n274 = case shown="\"KWP-2000\"" w877 {
                tunnel: w889 -> [w896 w907 w915]
                tunnel: w888 -> [w895 w905 w914]
                tunnel: [w900 w904 w913] -> w885
                tunnel: [w899 w903 w912] -> w883
                tunnel: w882 -> [w901 w908 w911]
                tunnel: w881 -> [w897 w906 w910]
                tunnel: [w898 w902 w909] -> w880
                frame "GMLAN", Default {
                  n275 = call "GMLAN DeviceControl.vi"("error in (no error)"=w901, "CPIDControlBytes"=w895, "CPID ID"=w896, "diag ref in"=w897) -> ("error out"=w900:errorcluster, "success?"=w899:bool, "diag ref out"=w898:T29)  [unwired: 5 in]
                }
                frame "KWP-2000" {
                  n276 = call <vilib>:"WriteDataByLocalIdentifier.vi"("data in"=w905, "error in (no error)"=w908, "local ID"=w907, "diag ref in"=w906) -> ("error out"=w904:errorcluster, "success?"=w903:bool, "diag ref out"=w902:T29)  [unwired: 5 in]
                }
                frame "UDS" {
                  n277 = call <vilib>:"UDS WriteDataByIdentifier.vi"("data in"=w914, "error in (no error)"=w911, "ID"=w915, "diag ref in"=w910) -> ("error out"=w913:errorcluster, "success?"=w912:bool, "diag ref out"=w909:T29)  [unwired: 5 in]
                }
              }
              n278 = call "Convert Boolean to DBL Array.vi"("Boolean"=w883) -> ("DBL Array"=w887:dbl[])  [unwired: 10 in]
              n279 = RT FIFO Write(0:w879, 1:w887) -> (8:w878:refnum<k33>, 11:w886:errorcluster)  [unwired: 3 in, 2 out]
              n280 = Merge Errors(w885, w886) -> (w884:errorcluster)
              n281 = in-place-cluster #20("Parameters.ChanRefs.ToVS.Status.Write to VS Engine FIFO"=w878, "ADCS Connection"=w880, "Parameters.Properties.CAN.Diagnostic Protocol"=w877) -> (w872:T1)
            }
          }
          frame Enabled {
            n282 = in-place {
              in-place-border: w920 -> [w946]
              in-place-border: w919 -> [w945]
              in-place-border: [w942] -> w918
              n283 = in-place-cluster #21(w917) -> ("Parameters.ChanRefs.ToVS.Status.Write to VS Engine FIFO"=w938:refnum<k33>, "ADCS Connection"=w940:T29, "Parameters.Properties.CAN.Diagnostic Protocol"=w936:T9, "Parameters.Properties.CPID Lookup"=w926:variant, "Parameters.ChanRefs.FromVS.CPIDs.Read from VS Engine FIFO"=w925:refnum<k33>, "Parameters.ChanRefs.FromVS.CPIDs.Pairs.Values"=w931:dbl[])
              n284 = Unflatten From String(type=u16 0, binary string=w945, error in (no error)=w946) -> (value=w932:u16, error out=w930:errorcluster)  [unwired: 2 in, 1 out]
              n285 = RT FIFO Read(0:w925, 1:w931, 3:w930) -> (8:w924:refnum<k33>, 9:w928:dbl[], 11:w929:errorcluster)  [unwired: 1 in, 2 out]
              n286 = call "IndexAndScaleGeneratedData.vi"("Lookup"=w926, "error in"=w929, "ID"=w932, "VS Data"=w928) -> ("error out"=w934:errorcluster, "Data"=w933:u8[], "VS Data"=w927:dbl[])  [unwired: 5 in]
              n287 = case shown="\"UDS\"" w936 {
                tunnel: w932 -> [w948 w959 w967]
                tunnel: w933 -> [w947 w957 w966]
                tunnel: [w952 w956 w965] -> w923
                tunnel: [w951 w955 w964] -> w941
                tunnel: w934 -> [w953 w960 w963]
                tunnel: w940 -> [w949 w958 w962]
                tunnel: [w950 w954 w961] -> w939
                frame "GMLAN", Default {
                  n288 = call "GMLAN DeviceControl.vi"("error in (no error)"=w953, "CPIDControlBytes"=w947, "CPID ID"=w948, "diag ref in"=w949) -> ("error out"=w952:errorcluster, "success?"=w951:bool, "diag ref out"=w950:T29)  [unwired: 5 in]
                }
                frame "KWP-2000" {
                  n289 = call <vilib>:"WriteDataByLocalIdentifier.vi"("data in"=w957, "error in (no error)"=w960, "local ID"=w959, "diag ref in"=w958) -> ("error out"=w956:errorcluster, "success?"=w955:bool, "diag ref out"=w954:T29)  [unwired: 5 in]
                }
                frame "UDS" {
                  n290 = call <vilib>:"UDS WriteDataByIdentifier.vi"("data in"=w966, "error in (no error)"=w963, "ID"=w967, "diag ref in"=w962) -> ("error out"=w965:errorcluster, "success?"=w964:bool, "diag ref out"=w961:T29)  [unwired: 5 in]
                }
              }
              n291 = call "Get Error Byte.vi"("error"=w923) -> ("error  out"=w922:errorcluster, "Error Byte"=w921:u8)  [unwired: 9 in]
              n292 = call "Convert Boolean to DBL Array.vi"("Error Code"=w921, "Boolean"=w941) -> ("DBL Array"=w944:dbl[])  [unwired: 9 in]
              n293 = RT FIFO Write(0:w938, 1:w944) -> (8:w937:refnum<k33>, 11:w943:errorcluster)  [unwired: 3 in, 2 out]
              n294 = Merge Errors(w922, w943) -> (w942:errorcluster)
              n295 = in-place-cluster #21("Parameters.ChanRefs.ToVS.Status.Write to VS Engine FIFO"=w937, "ADCS Connection"=w939, "Parameters.Properties.CAN.Diagnostic Protocol"=w936, "Parameters.Properties.CPID Lookup"=w926, "Parameters.ChanRefs.FromVS.CPIDs.Read from VS Engine FIFO"=w924, "Parameters.ChanRefs.FromVS.CPIDs.Pairs.Values"=w927) -> (w916:T1)
            }
          }
        }
      }
      frame "ReadPIDOnDemand", "ReadPIDsOnDemand" {
        n296 = in-place {
          in-place-border: w973 -> [w991]
          in-place-border: w972 -> [w990]
          in-place-border: w971 -> [w989]
          in-place-border: [w988] -> w970
          n297 = in-place-cluster #22(w969) -> ("Parameters.ChanRefs.ToVS.Status.Write to VS Engine FIFO"=w987:refnum<k33>, "Parameters.ChanRefs.ToVS.PIDs.Write to VS Engine FIFO"=w986:refnum<k33>, "ADCS Connection"=w981:T29, "Parameters.ChanRefs.ToVS.PIDs.Pairs.Values"=w985:dbl[], "Parameters.Properties.PID Lookup"=w983:variant, "Parameters.Properties.PIDs"=w982:T13[], "XNETEngine (GMLAN)"=w978:T32, "Parameters.Properties.CAN.Diagnostic Protocol"=w979:T9)
          n298 = case shown="\"ReadPIDsOnDemand\", Default" w989 {
            tunnel: w982 -> [_ w1050]
            tunnel: [w1042 w1049] -> w992
            tunnel: w991 -> [w1047 w1048]
            tunnel: [w1046 w1048] -> w993
            tunnel: w990 -> [w1044 _]
            frame "ReadPIDOnDemand" {
              n299 = Unflatten From String(type=u16 0 ("ID"), binary string=w1044, error in (no error)=w1047) -> (value=w1043:u16, error out=w1046:errorcluster)  [unwired: 2 in, 1 out]
              n300 = Build Array(w1043) -> (w1042:u16[])
            }
            frame "ReadPIDsOnDemand", Default {
              n301 = for {
                tunnel: w1050 -> [w1052] mode=indexing
                tunnel: [w1051] -> w1049 mode=indexing
                n302 = Unbundle By Name(w1052) -> ("ID"=w1051:u32)
              }
            }
          }
          n303 = case shown="\"KWP-2000\", \"UDS\"" w979 {
            selector: w979 -> [_ w1022]
            tunnel: [w1005 w1031] -> w977
            tunnel: [w1000 w1030] -> w996
            tunnel: w993 -> [w1006 w1029]
            tunnel: w992 -> [w1003 w1028]
            tunnel: w985 -> [w1001 w1027]
            tunnel: [w1001 w1026] -> w984
            tunnel: w983 -> [_ w1025]
            tunnel: w981 -> [w1004 w1024]
            tunnel: [w1002 w1023] -> w980
            tunnel: w978 -> [w999 _]
            frame "GMLAN" {
              n304 = for {
                shift-right: [w1017] -> w1011
                shift-left: w1006 -> [w1021]
                shift-right: [w1019] -> w1002
                shift-left: w1004 -> [w1020]
                tunnel: w1003 -> [w1012] mode=indexing
                tunnel: [w1018] -> w1000 mode=indexing
                tunnel: [w1015] -> w1007 mode=indexing
                stop <- w1017 stop-if-true
                n305 = call "GMLAN ReadDataByParameterIdentifier.vi"("error in (no error)"=w1021, "Parameter ID (PID)"=w1012, "diag ref in"=w1020) -> ("error out"=w1017:errorcluster, "success?"=w1018:bool, "data out"=w1016:u8[], "diag ref out"=w1019:T29)  [unwired: 5 in]
                n306 = call "Initialize Raw XNET Frame.vi"("Data"=w1016, "identifier"=w1012) -> ("Raw Frame"=w1013:u8[])  [unwired: 9 in]
                n307 = Bundle By Name(cluster=T42 {"ID"=0, "Raw Frame"=[]}, "ID"=w1012, "Raw Frame"=w1013) -> (w1015:T42)
              }
              n308 = Flatten To String(anything=w1007, error in (no error)=w1011) -> (data string=w1008:string, error out=w1010:errorcluster)  [unwired: 2 in, 1 out]
              n309 = call <vilib>:"Send Local Message.vi"("message queue in"=w999, "message name"="UpdatePIDsOnDemand" ("Message Name"), "message value"=w1008, "error in"=w1010) -> ("error out"=w1005:errorcluster)  [unwired: 9 in, 2 out]
            }
            frame "KWP-2000", "UDS" {
              n310 = for {
                shift-right: [w1039] -> w1031
                shift-left: w1029 -> [w1041]
                shift-right: [w1033] -> w1023
                shift-left: w1024 -> [w1037]
                shift-right: [w1032] -> w1026
                shift-left: w1027 -> [w1036]
                tunnel: w1025 -> [w1034]
                tunnel: w1028 -> [w1035] mode=indexing
                tunnel: [w1040] -> w1030 mode=indexing
                tunnel: w1022 -> [w1038]
                stop <- w1039 stop-if-true
                n311 = call "Read PIDDIDs.vi"("Diagnostic Protocol"=w1038, "ID"=w1035, "error in (no error)"=w1041, "Lookup"=w1034, "Values in"=w1036, "ADCS Connection"=w1037) -> ("error out"=w1039:errorcluster, "success?"=w1040:bool, "Values out"=w1032:dbl[], "diag ref out"=w1033:T29)  [unwired: 2 in]
              }
            }
          }
          n312 = And Array Elements(Boolean array=w996) -> (logical AND=w994:bool)
          n313 = call "Get Error Byte.vi"("error"=w977) -> ("error  out"=w976:errorcluster, "Error Byte"=w975:u8)  [unwired: 9 in]
          n314 = call "Convert Boolean to DBL Array.vi"("Error Code"=w975, "Boolean"=w994) -> ("DBL Array"=w995:dbl[])  [unwired: 9 in]
          n315 = RT FIFO Write(0:w987, 1:w995) -> (11:w998:errorcluster)  [unwired: 3 in, 3 out]
          n316 = Merge Errors(w976, w998) -> (w997:errorcluster)
          n317 = RT FIFO Write(0:w986, 1:w984, 3:w997) -> (11:w988:errorcluster)  [unwired: 2 in, 3 out]
          n318 = in-place-cluster #22("Parameters.ChanRefs.ToVS.Status.Write to VS Engine FIFO"=w987, "Parameters.ChanRefs.ToVS.PIDs.Write to VS Engine FIFO"=w986, "ADCS Connection"=w980, "Parameters.ChanRefs.ToVS.PIDs.Pairs.Values"=w984, "Parameters.Properties.PID Lookup"=w983, "Parameters.Properties.PIDs"=w982, "XNETEngine (GMLAN)"=w978, "Parameters.Properties.CAN.Diagnostic Protocol"=w979) -> (w968:T1)
        }
      }
      frame "ReadDID", "ReadDIDs" {
        n319 = in-place {
          in-place-border: w1057 -> [w1075]
          in-place-border: w1056 -> [w1074]
          in-place-border: w1058 -> [w1073]
          in-place-border: [w1072] -> w1055
          n320 = in-place-cluster #23(w1054) -> ("Parameters.ChanRefs.ToVS.Status.Write to VS Engine FIFO"=w1071:refnum<k33>, "Parameters.ChanRefs.ToVS.DIDs.Write to VS Engine FIFO"=w1070:refnum<k33>, "ADCS Connection"=w1065:T29, "Parameters.ChanRefs.ToVS.DIDs.Pairs.Values"=w1069:dbl[], "Parameters.Properties.DID Lookup"=w1067:variant, "Parameters.Properties.DIDs"=w1066:T13[], "Parameters.Properties.CAN.Diagnostic Protocol"=w1063:T9)
          n321 = case shown="\"ReadDID\"" w1073 {
            tunnel: w1066 -> [_ w1091]
            tunnel: [w1083 w1090] -> w1076
            tunnel: w1075 -> [w1088 w1089]
            tunnel: [w1087 w1089] -> w1077
            tunnel: w1074 -> [w1085 _]
            frame "ReadDID" {
              n322 = Unflatten From String(type=u16 0 ("ID"), binary string=w1085, error in (no error)=w1088) -> (value=w1084:u16, error out=w1087:errorcluster)  [unwired: 2 in, 1 out]
              n323 = Build Array(w1084) -> (w1083:u16[])
            }
            frame "ReadDIDs", Default {
              n324 = for {
                tunnel: w1091 -> [w1093] mode=indexing
                tunnel: [w1092] -> w1090 mode=indexing
                n325 = Unbundle By Name(w1093) -> ("ID"=w1092:u32)
              }
            }
          }
          n326 = for {
            shift-right: [w1101] -> w1062
            shift-left: w1077 -> [w1103]
            shift-right: [w1095] -> w1064
            shift-left: w1065 -> [w1099]
            shift-right: [w1094] -> w1068
            shift-left: w1069 -> [w1098]
            tunnel: w1067 -> [w1096]
            tunnel: w1076 -> [w1097] mode=indexing
            tunnel: [w1102] -> w1080 mode=indexing
            tunnel: w1063 -> [w1100]
            stop <- w1101 stop-if-true
            n327 = call "Read PIDDIDs.vi"("Diagnostic Protocol"=w1100, "ID"=w1097, "error in (no error)"=w1103, "Lookup"=w1096, "Values in"=w1098, "ADCS Connection"=w1099) -> ("error out"=w1101:errorcluster, "success?"=w1102:bool, "Values out"=w1094:dbl[], "diag ref out"=w1095:T29)  [unwired: 2 in]
          }
          n328 = And Array Elements(Boolean array=w1080) -> (logical AND=w1078:bool)
          n329 = call "Get Error Byte.vi"("error"=w1062) -> ("error  out"=w1061:errorcluster, "Error Byte"=w1060:u8)  [unwired: 9 in]
          n330 = call "Convert Boolean to DBL Array.vi"("Error Code"=w1060, "Boolean"=w1078) -> ("DBL Array"=w1079:dbl[])  [unwired: 9 in]
          n331 = RT FIFO Write(0:w1071, 1:w1079) -> (11:w1082:errorcluster)  [unwired: 3 in, 3 out]
          n332 = Merge Errors(w1061, w1082) -> (w1081:errorcluster)
          n333 = in-place-cluster #23("Parameters.ChanRefs.ToVS.Status.Write to VS Engine FIFO"=w1071, "Parameters.ChanRefs.ToVS.DIDs.Write to VS Engine FIFO"=w1070, "ADCS Connection"=w1064, "Parameters.ChanRefs.ToVS.DIDs.Pairs.Values"=w1068, "Parameters.Properties.DID Lookup"=w1067, "Parameters.Properties.DIDs"=w1066, "Parameters.Properties.CAN.Diagnostic Protocol"=w1063) -> (w1053:T1)
          n334 = RT FIFO Write(0:w1070, 1:w1068, 3:w1081) -> (11:w1072:errorcluster)  [unwired: 2 in, 3 out]
        }
      }
      frame "ECUReset" {
        n335 = in-place {
          in-place-border: w1108 -> [w1120]
          in-place-border: [w1119] -> w1107
          in-place-border: w1106 -> [w1118]
          n336 = in-place-cluster #24(w1105) -> ("Parameters.ChanRefs.ToVS.Status.Write to VS Engine FIFO"=w1115:refnum<k33>, "Parameters.Properties.CAN.Diagnostic Protocol"=w1113:T9, "ADCS Connection"=w1117:T29)
          n337 = Unflatten From String(type=u8 0 ("ID"), binary string=w1118, error in (no error)=w1120) -> (value=w1125:u8, error out=w1124:errorcluster)  [unwired: 2 in, 1 out]
          n338 = case shown="\"UDS\"" w1113 {
            tunnel: [FALSE ("success?") w1133 w1141] -> w1126
            tunnel: [w1128 w1134 w1140] -> w1112
            tunnel: w1125 -> [_ w1130 w1139]
            tunnel: w1124 -> [w1128 w1135 w1138]
            tunnel: w1117 -> [w1129 w1131 w1137]
            tunnel: [w1129 w1132 w1136] -> w1116
            frame "GMLAN" {
            }
            frame "KWP-2000" {
              n339 = call <vilib>:"ECUReset.vi"("error in (no error)"=w1135, "mode"=w1130, "diag ref in"=w1131) -> ("error out"=w1134:errorcluster, "success?"=w1133:bool, "diag ref out"=w1132:T29)  [unwired: 6 in]
            }
            frame "UDS" {
              n340 = call <vilib>:"UDS ECUReset.vi"("error in (no error)"=w1138, "mode"=w1139, "diag ref in"=w1137) -> ("error out"=w1140:errorcluster, "success?"=w1141:bool, "diag ref out"=w1136:T29)  [unwired: 5 in, 1 out]
            }
          }
          n341 = call "Get Error Byte.vi"("error"=w1112) -> ("error  out"=w1111:errorcluster, "Error Byte"=w1110:u8)  [unwired: 9 in]
          n342 = call "Convert Boolean to DBL Array.vi"("Error Code"=w1110, "Boolean"=w1126) -> ("DBL Array"=w1123:dbl[])  [unwired: 9 in]
          n343 = RT FIFO Write(0:w1115, 1:w1123) -> (8:w1114:refnum<k33>, 11:w1122:errorcluster)  [unwired: 3 in, 2 out]
          n344 = Merge Errors(w1111, w1122) -> (w1119:errorcluster)
          n345 = in-place-cluster #24("Parameters.ChanRefs.ToVS.Status.Write to VS Engine FIFO"=w1114, "Parameters.Properties.CAN.Diagnostic Protocol"=w1113, "ADCS Connection"=w1116) -> (w1104:T1)
        }
      }
      frame "<--------------- TCP ONLY --------------->" {
      }
      frame "PassThru" {
        n346 = in-place {
          in-place-border: w1151 -> [w1174]
          in-place-border: [w1173] -> w1150
          in-place-border: w1149 -> [w1166]
          in-place-border: w1148 -> [w1163]
          in-place-border: w1147 -> [w1162]
          n347 = in-place-cluster #25(w1146) -> ("ADCS Connection"=w1157:T29)
          n348 = Unflatten From String(type=cluster{"cmd":u8[], "require response?":bool} {"cmd"=[], "require response?"=TRUE}, binary string=w1163, error in (no error)=w1162) -> (value=w1160:cluster{"cmd":u8[], "require response?":bool}, error out=w1153:errorcluster)  [unwired: 2 in, 1 out]
          n349 = Unbundle By Name(w1160) -> ("require response?"=w1158:bool, "cmd"=w1159:u8[])
          n350 = call <vilib>:"Diagnostic Service.vi"("error source"="Diagnostic Service.vi", "error in (no error)"=w1153, "data in"=w1159, "require response?"=w1158, "diag ref in"=w1157) -> ("error out"=w1154:errorcluster, "data out"=w1170:u8[], "error code"=w1171:u8, "diag ref out"=w1156:T29)  [unwired: 1 in, 2 out]
          n351 = global read "GUID Lookup.vi" "ResponseQKey"() -> (w1178:string)
          n352 = Unbundle By Name(w1174) -> ("attributes"=w1175:T47)
          n353 = Bundle By Name(cluster=T43 {"resp"=[], "error code"=0, "error out"={"status"=FALSE, "code"=0, "source"=""}}, "error code"=w1171, "resp"=w1170, "error out"=w1154) -> (w1168:T43)
          n354 = call <vilib>:"Index.vi"("key"=w1178, "array in"=w1175) -> ("value"=w1177:string)  [unwired: 3 in, 2 out]
          n355 = Flatten To String(anything=w1168, error in (no error)=w1153) -> (data string=w1167:string, error out=w1169:errorcluster)  [unwired: 2 in, 1 out]
          n356 = Concatenate Strings(w1166, "Response" ("string")) -> (w1164:string)
          n357 = Empty String/Path?(string/path=w1177) -> (empty?=w1176:bool)
          n358 = case shown="False" w1176 {
            tunnel: w1169 -> [w1183 w1184]
            tunnel: [w1182 w1184] -> w1173
            tunnel: w1177 -> [w1181 _]
            tunnel: w1164 -> [w1180 _]
            tunnel: w1167 -> [w1179 _]
            frame False {
              n359 = call <vilib>:"Send Local Message.vi"("receiver process (\"\" - local)"=w1181, "message name"=w1180, "message value"=w1179, "error in"=w1183) -> ("error out"=w1182:errorcluster)  [unwired: 9 in, 2 out]
            }
            frame True {
            }
          }
          n360 = in-place-cluster #25("ADCS Connection"=w1156) -> (w1145:T1)
        }
      }
      frame "<--------------- UDS/KWP ONLY --------------->" {
      }
      frame "ReadMemory" {
        n361 = in-place {
          in-place-border: w1192 -> [w1209]
          in-place-border: [w1210] -> w1191
          in-place-border: w1190 -> [w1208]
          n362 = in-place-cluster #26(w1189) -> ("Parameters.ChanRefs.ToVS.Status.Write to VS Engine FIFO"=w1214:refnum<k33>, "Parameters.Properties.CAN.Diagnostic Protocol"=w1217:T9, "Parameters.Properties.Memory.Read Lookup"=w1197:variant, "Parameters.ChanRefs.ToVS.ReadMemory.Write to VS Engine FIFO"=w1203:refnum<k33>, "Parameters.ChanRefs.ToVS.ReadMemory.Pairs.Values"=w1205:dbl[], "ADCS Connection"=w1218:T29)
          n363 = Unflatten From String(type=u32 0 ("ID"), binary string=w1208, error in (no error)=w1209) -> (value=w1199:u32, error out=w1198:errorcluster)  [unwired: 2 in, 1 out]
          n364 = case shown="\"KWP-2000\"" w1217 {
            tunnel: [w1228 w1234 w1240] -> w1206
            tunnel: [w1230 w1236 w1239] -> w1216
            tunnel: w1198 -> [w1220 w1235 w1240]
            tunnel: w1218 -> [w1231 w1237 w1239]
            tunnel: [w1227 w1233 _] -> w1212
            tunnel: w1199 -> [w1222 w1238 _]
            tunnel: [w1229 w1232 _] -> w1207
            tunnel: w1197 -> [w1223 _ _]
            frame "KWP-2000" {
              n365 = Type Cast(x=w1222) -> (*(type *) &x=w1226:string)  [unwired: 1 in]
              n366 = Get Variant Attribute(Variant=w1223, name=w1226, default value (empty Variant)=T44 {"Offset"=0, "Length"=0, "ByteLength"=0} ("cluster"), error in=w1220) -> (value=w1224:T44, error out=w1219:errorcluster)  [unwired: 2 out]
              n367 = Unbundle By Name(w1224) -> ("ByteLength"=w1221:u16)
              n368 = call <vilib>:"ReadMemoryByAddress.vi"("error in (no error)"=w1219, "size"=w1221, "address"=w1222, "diag ref in"=w1231) -> ("error out"=w1228:errorcluster, "success?"=w1227:bool, "data out"=w1229:u8[], "diag ref out"=w1230:T29)  [unwired: 4 in]
            }
            frame "UDS" {
              n369 = call <vilib>:"UDS ReadDataByIdentifier.vi"("error in (no error)"=w1235, "ID"=w1238, "diag ref in"=w1237) -> ("error out"=w1234:errorcluster, "success?"=w1233:bool, "data out"=w1232:u8[], "diag ref out"=w1236:T29)  [unwired: 5 in]
            }
            frame "GMLAN" {
            }
          }
          n370 = call "ScaleAndReplaceAcquiredData.vi"("Lookup"=w1197, "error in (no error)"=w1206, "Unscaled Data"=w1207, "ID"=w1199, "VS Data"=w1205) -> ("error out"=w1204:errorcluster, "VS Data"=w1201:dbl[])  [unwired: 5 in]
          n371 = RT FIFO Write(0:w1203, 1:w1201, 3:w1204) -> (8:w1202:refnum<k33>, 11:w1196:errorcluster)  [unwired: 2 in, 2 out]
          n372 = call "Get Error Byte.vi"("error"=w1196) -> ("error  out"=w1195:errorcluster, "Error Byte"=w1194:u8)  [unwired: 9 in]
          n373 = call "Convert Boolean to DBL Array.vi"("Error Code"=w1194, "Boolean"=w1212) -> ("DBL Array"=w1215:dbl[])  [unwired: 9 in]
          n374 = RT FIFO Write(0:w1214, 1:w1215) -> (8:w1213:refnum<k33>, 11:w1211:errorcluster)  [unwired: 3 in, 2 out]
          n375 = Merge Errors(w1195, w1211) -> (w1210:errorcluster)
          n376 = in-place-cluster #26("Parameters.ChanRefs.ToVS.Status.Write to VS Engine FIFO"=w1213, "Parameters.Properties.CAN.Diagnostic Protocol"=w1217, "Parameters.Properties.Memory.Read Lookup"=w1197, "Parameters.ChanRefs.ToVS.ReadMemory.Write to VS Engine FIFO"=w1202, "Parameters.ChanRefs.ToVS.ReadMemory.Pairs.Values"=w1201, "ADCS Connection"=w1216) -> (w1188:T1)
        }
      }
      frame "WriteMemory" {
        n377 = in-place {
          in-place-border: w1245 -> [w1263]
          in-place-border: [w1264] -> w1244
          in-place-border: w1243 -> [w1262]
          n378 = in-place-cluster #27(w1242) -> ("Parameters.ChanRefs.ToVS.Status.Write to VS Engine FIFO"=w1268:refnum<k33>, "Parameters.Properties.CAN.Diagnostic Protocol"=w1271:T9, "ADCS Connection"=w1272:T29, "Parameters.Properties.Memory.Write Lookup"=w1252:variant, "Parameters.ChanRefs.FromVS.WriteMemory.Read from VS Engine FIFO"=w1255:refnum<k33>, "Parameters.ChanRefs.FromVS.WriteMemory.Pairs.Values"=w1256:dbl[])
          n379 = Unflatten From String(type=u32 0 ("ID"), binary string=w1262, error in (no error)=w1263) -> (value=w1250:u32, error out=w1259:errorcluster)  [unwired: 2 in, 1 out]
          n380 = RT FIFO Read(0:w1255, 1:w1256, 3:w1259) -> (8:w1254:refnum<k33>, 9:w1260:dbl[], 11:w1261:errorcluster)  [unwired: 1 in, 2 out]
          n381 = call "IndexAndScaleGeneratedData.vi"("Lookup"=w1252, "error in"=w1261, "ID"=w1250, "VS Data"=w1260) -> ("error out"=w1258:errorcluster, "Data"=w1257:u8[], "VS Data"=w1253:dbl[])  [unwired: 5 in]
          n382 = case shown="\"UDS\"" w1271 {
            tunnel: [w1278 w1286 w1289] -> w1249
            tunnel: [w1276 w1284 w1288] -> w1270
            tunnel: w1258 -> [w1279 w1287 w1289]
            tunnel: w1272 -> [w1280 w1282 w1288]
            tunnel: [w1277 w1285 _] -> w1266
            tunnel: w1250 -> [w1275 w1283 _]
            tunnel: w1257 -> [w1273 w1281 _]
            frame "KWP-2000" {
              n383 = Array Size(array=w1273) -> (size(s)=w1274:i32)
              n384 = call <vilib>:"WriteMemoryByAddress.vi"("data in"=w1273, "error in (no error)"=w1279, "size"=w1274, "address"=w1275, "diag ref in"=w1280) -> ("error out"=w1278:errorcluster, "success?"=w1277:bool, "diag ref out"=w1276:T29)  [unwired: 4 in]
            }
            frame "UDS" {
              n385 = call <vilib>:"UDS WriteDataByIdentifier.vi"("data in"=w1281, "error in (no error)"=w1287, "ID"=w1283, "diag ref in"=w1282) -> ("error out"=w1286:errorcluster, "success?"=w1285:bool, "diag ref out"=w1284:T29)  [unwired: 5 in]
            }
            frame "GMLAN" {
            }
          }
          n386 = call "Get Error Byte.vi"("error"=w1249) -> ("error  out"=w1248:errorcluster, "Error Byte"=w1247:u8)  [unwired: 9 in]
          n387 = call "Convert Boolean to DBL Array.vi"("Error Code"=w1247, "Boolean"=w1266) -> ("DBL Array"=w1269:dbl[])  [unwired: 9 in]
          n388 = RT FIFO Write(0:w1268, 1:w1269) -> (8:w1267:refnum<k33>, 11:w1265:errorcluster)  [unwired: 3 in, 2 out]
          n389 = Merge Errors(w1248, w1265) -> (w1264:errorcluster)
          n390 = in-place-cluster #27("Parameters.ChanRefs.ToVS.Status.Write to VS Engine FIFO"=w1267, "Parameters.Properties.CAN.Diagnostic Protocol"=w1271, "ADCS Connection"=w1270, "Parameters.Properties.Memory.Write Lookup"=w1252, "Parameters.ChanRefs.FromVS.WriteMemory.Read from VS Engine FIFO"=w1254, "Parameters.ChanRefs.FromVS.WriteMemory.Pairs.Values"=w1253) -> (w1241:T1)
        }
      }
      frame "InputOutputControl" {
        n391 = disable-structure shown="Enabled" {
          disable-tunnel: w1294 -> [w1333 w1358]
          disable-tunnel: w1293 -> [w1332 w1356]
          disable-tunnel: [w1331 w1357] -> w1292
          disable-tunnel: w1291 -> [_ w1355]
          disable-tunnel: [_ w1354] -> w1290
          frame Disabled {
            n392 = Unflatten From String(type=u16[] [], binary string=w1332, error in (no error)=w1333) -> (value=w1319:u16[], error out=w1306:errorcluster)  [unwired: 2 in, 1 out]
            n393 = Index Array(array=w1319) -> (element #1=w1302:u16, element #2=w1316:u16)  [unwired: 2 in]
            n394 = global read "GUID Lookup.vi" "LookupTableConvertPrefix"() -> (w1310:string)
            n395 = Type Cast(x=w1302) -> (*(type *) &x=w1308:string)  [unwired: 1 in]
            n396 = RT FIFO Read() -> (9:w1296:dbl[])  [unwired: 4 in, 4 out]
            n397 = Get Variant Attribute(name=w1308, default value (empty Variant)=T44 {"Offset"=0, "Length"=0, "ByteLength"=0} ("cluster"), error in=w1306) -> (duplicate Variant=w1307:variant, value=w1305:T44, error out=w1309:errorcluster)  [unwired: 1 in, 1 out]
            n398 = Unbundle By Name(w1305) -> ("Offset"=w1304:i32, "Length"=w1303:i32)
            n399 = Concatenate Strings(w1310, w1308) -> (w1311:string)
            n400 = Get Variant Attribute(Variant=w1307, name=w1311, default value (empty Variant)=refnum<k21> refnum ("DID Conversion"), error in=w1309) -> (value=w1300:refnum<k21>, error out=w1298:errorcluster)  [unwired: 2 out]
            n401 = Array Subset(array=w1296, index=w1304, length=w1303) -> (w1301:dbl[])
            n402 = Type Cast(x=w1302) -> (*(type *) &x=w1322:string)  [unwired: 1 in]
            n403 = call-poly <vilib>:"XNET Convert.vi"("session in"=w1300, "signal data"=w1301, "error in (no error)"=w1298) -> ("frame data"=w1299:u8[], "error out"=w1297:errorcluster)  [unwired: 10 in, 1 out]
            n404 = call <vilib>:"UDS InputOutputControlByIdentifier.vi"("data in"=w1299, "error in (no error)"=w1297, "mode"=w1316, "ID"=w1302) -> ("error out"=w1318:errorcluster, "success?"=w1314:bool, "data out"=w1315:u8[], "diag ref out"=w1317:T29)  [unwired: 4 in]
            n405 = call "Initialize Raw XNET Frame.vi"("Data"=w1315, "identifier"=w1302) -> ("Raw Frame"=w1324:u8[])  [unwired: 9 in]
            n406 = global read "GUID Lookup.vi" "LookupTableConvertPrefix"() -> (w1329:string)
            n407 = Concatenate Strings(w1329, w1322) -> (w1327:string)
            n408 = Get Variant Attribute(name=w1327, default value (empty Variant)=refnum<k21> refnum ("DID Conversion"), error in=w1318) -> (duplicate Variant=w1323:variant, found=w1321:bool, value=w1325:refnum<k21>, error out=w1328:errorcluster)  [unwired: 1 in]
            n409 = case shown="False" w1321 {
              tunnel: [_ w1351] -> w1330
              tunnel: [w1339 w1349] -> w1335
              tunnel: w1328 -> [w1339 w1348]
              tunnel: w1325 -> [_ w1347]
              tunnel: w1324 -> [_ w1346]
              tunnel: w1323 -> [_ w1345]
              tunnel: w1322 -> [_ w1344]
              tunnel: w1317 -> [w1338 w1341]
              tunnel: [w1338 w1341] -> _
              frame False {
                n410 = disable-structure shown="Default" {
                  frame condition #0 {
                    # "DLE NOTE - ERROR!!"
                    n411 = call <vilib>:"NI VeriStand - Print Debug String.vi"("Message"="Debug Error-DID Scaling Note Found!!" ("Debug String")) -> ()  [unwired: 10 in, 1 out]
                  }
                  frame condition #1 (active) {
                  }
                }
              }
              frame True {
                # "Scale PID"
                n412 = call-poly <vilib>:"XNET Convert.vi"("session in"=w1347, "frame data"=w1346, "error in (no error)"=w1348) -> ("signal data"=w1342:dbl[], "error out"=w1350:errorcluster)  [unwired: 10 in, 1 out]
                n413 = Get Variant Attribute(Variant=w1345, name=w1344, default value (empty Variant)=T44 {"Offset"=0, "Length"=0, "ByteLength"=0} ("cluster"), error in=w1350) -> (value=w1353:T44, error out=w1349:errorcluster)  [unwired: 2 out]
                n414 = Unbundle By Name(w1353) -> ("Offset"=w1343:i32)
                n415 = Replace Array Subset(new element=w1342, index=w1343) -> (w1351:dbl[])  [unwired: 1 in]
              }
            }
            n416 = call "Convert Boolean to DBL Array.vi"("Boolean"=w1314) -> ("DBL Array"=w1334:dbl[])  [unwired: 10 in]
            n417 = RT FIFO Write(1:w1334) -> (11:w1337:errorcluster)  [unwired: 4 in, 3 out]
            n418 = Merge Errors(w1335, w1337) -> (w1336:errorcluster)
            n419 = RT FIFO Write(1:w1330, 3:w1336) -> (11:w1331:errorcluster)  [unwired: 3 in, 3 out]
          }
          frame Enabled {
            n420 = in-place {
              in-place-border: w1358 -> [w1385]
              in-place-border: [w1386] -> w1357
              in-place-border: w1356 -> [w1384]
              n421 = in-place-cluster #28(w1355) -> ("Parameters.ChanRefs.ToVS.Status.Write to VS Engine FIFO"=w1390:refnum<k33>, "Parameters.Properties.CAN.Diagnostic Protocol"=w1393:T9, "Parameters.Properties.IO.Resp Lookup"=w1371:variant, "Parameters.ChanRefs.ToVS.IO.Resp.Write to VS Engine FIFO"=w1368:refnum<k33>, "Parameters.ChanRefs.ToVS.IO.Resp.Pairs.Values"=w1370:dbl[], "ADCS Connection"=w1394:T29, "Parameters.Properties.IO.Cmd Lookup"=w1374:variant, "Parameters.ChanRefs.FromVS.IO.Cmd.Read from VS Engine FIFO"=w1377:refnum<k33>, "Parameters.ChanRefs.FromVS.IO.Cmd.Pairs.Values"=w1378:dbl[])
              n422 = Unflatten From String(type=T45 {"ID"=0, "Mode"=0}, binary string=w1384, error in (no error)=w1385) -> (value=w1364:T45, error out=w1381:errorcluster)  [unwired: 2 in, 1 out]
              n423 = Unbundle By Name(w1364) -> ("ID"=w1363:u16, "Mode"=w1362:u8)
              n424 = RT FIFO Read(0:w1377, 1:w1378, 3:w1381) -> (8:w1376:refnum<k33>, 9:w1382:dbl[], 11:w1383:errorcluster)  [unwired: 1 in, 2 out]
              n425 = call "IndexAndScaleGeneratedData.vi"("Lookup"=w1374, "error in"=w1383, "ID"=w1363, "VS Data"=w1382) -> ("error out"=w1380:errorcluster, "Data"=w1379:u8[], "VS Data"=w1375:dbl[])  [unwired: 5 in]
              n426 = case shown="\"KWP-2000\"" w1393 {
                tunnel: [w1403 w1411 w1414] -> w1372
                tunnel: [w1402 w1406 w1413] -> w1392
                tunnel: w1380 -> [w1400 w1412 w1414]
                tunnel: w1394 -> [w1401 w1409 w1413]
                tunnel: [w1399 w1404 _] -> w1388
                tunnel: w1363 -> [w1398 w1410 _]
                tunnel: w1379 -> [w1397 w1408 _]
                tunnel: [w1396 w1405 _] -> w1373
                tunnel: w1362 -> [w1395 w1407 _]
                frame "KWP-2000" {
                  n427 = call <vilib>:"InputOutputControlByLocalIdentifier.vi"("data in"=w1397, "error in (no error)"=w1400, "mode"=w1395, "local ID"=w1398, "diag ref in"=w1401) -> ("error out"=w1403:errorcluster, "success?"=w1399:bool, "data out"=w1396:u8[], "diag ref out"=w1402:T29)  [unwired: 3 in]
                }
                frame "UDS" {
                  n428 = call <vilib>:"UDS InputOutputControlByIdentifier.vi"("data in"=w1408, "error in (no error)"=w1412, "mode"=w1407, "ID"=w1410, "diag ref in"=w1409) -> ("error out"=w1411:errorcluster, "success?"=w1404:bool, "data out"=w1405:u8[], "diag ref out"=w1406:T29)  [unwired: 3 in]
                }
                frame "GMLAN" {
                }
              }
              n429 = call "ScaleAndReplaceAcquiredData.vi"("Lookup"=w1371, "error in (no error)"=w1372, "Unscaled Data"=w1373, "ID"=w1363, "VS Data"=w1370) -> ("error out"=w1369:errorcluster, "VS Data"=w1366:dbl[])  [unwired: 5 in]
              n430 = RT FIFO Write(0:w1368, 1:w1366, 3:w1369) -> (8:w1367:refnum<k33>, 11:w1361:errorcluster)  [unwired: 2 in, 2 out]
              n431 = call "Get Error Byte.vi"("error"=w1361) -> ("error  out"=w1360:errorcluster, "Error Byte"=w1359:u8)  [unwired: 9 in]
              n432 = call "Convert Boolean to DBL Array.vi"("Error Code"=w1359, "Boolean"=w1388) -> ("DBL Array"=w1391:dbl[])  [unwired: 9 in]
              n433 = RT FIFO Write(0:w1390, 1:w1391) -> (8:w1389:refnum<k33>, 11:w1387:errorcluster)  [unwired: 3 in, 2 out]
              n434 = Merge Errors(w1360, w1387) -> (w1386:errorcluster)
              n435 = in-place-cluster #28("Parameters.ChanRefs.ToVS.Status.Write to VS Engine FIFO"=w1389, "Parameters.Properties.CAN.Diagnostic Protocol"=w1393, "Parameters.Properties.IO.Resp Lookup"=w1371, "Parameters.ChanRefs.ToVS.IO.Resp.Write to VS Engine FIFO"=w1367, "Parameters.ChanRefs.ToVS.IO.Resp.Pairs.Values"=w1366, "ADCS Connection"=w1392, "Parameters.Properties.IO.Cmd Lookup"=w1374, "Parameters.ChanRefs.FromVS.IO.Cmd.Read from VS Engine FIFO"=w1376, "Parameters.ChanRefs.FromVS.IO.Cmd.Pairs.Values"=w1375) -> (w1354:T1)
            }
          }
        }
      }
      frame "StartRoutine" {
        n436 = in-place {
          in-place-border: w1419 -> [w1445]
          in-place-border: [w1446] -> w1418
          in-place-border: w1415 -> [w1443]
          n437 = in-place-cluster #29(w1417) -> ("Parameters.ChanRefs.ToVS.Status.Write to VS Engine FIFO"=w1450:refnum<k33>, "Parameters.Properties.CAN.Diagnostic Protocol"=w1453:T9, "Routine.Start.Resp Lookup"=w1429:variant, "Parameters.ChanRefs.ToVS.Routine.Start.Write to VS Engine FIFO"=w1426:refnum<k33>, "Parameters.ChanRefs.ToVS.Routine.Start.Pairs.Values"=w1428:dbl[], "ADCS Connection"=w1454:T29, "Routine.Start.Cmd Lookup"=w1433:variant, "Parameters.ChanRefs.FromVS.Routine.Start.Read from VS Engine FIFO"=w1436:refnum<k33>, "Parameters.ChanRefs.FromVS.Routine.Start.Pairs.Values"=w1437:dbl[])
          n438 = Unflatten From String(type=u16 0, binary string=w1443, error in (no error)=w1445) -> (value=w1431:u16, error out=w1440:errorcluster)  [unwired: 2 in, 1 out]
          n439 = RT FIFO Read(0:w1436, 1:w1437, 3:w1440) -> (8:w1435:refnum<k33>, 9:w1441:dbl[], 11:w1442:errorcluster)  [unwired: 1 in, 2 out]
          n440 = call "IndexAndScaleGeneratedData.vi"("Lookup"=w1433, "error in"=w1442, "ID"=w1431, "VS Data"=w1441) -> ("error out"=w1439:errorcluster, "Data"=w1438:u8[], "VS Data"=w1434:dbl[])  [unwired: 5 in]
          n441 = case shown="\"UDS\"" w1453 {
            tunnel: [w1462 w1471 w1473] -> w1430
            tunnel: [w1461 w1469 w1472] -> w1452
            tunnel: w1439 -> [w1459 w1468 w1473]
            tunnel: w1454 -> [w1460 w1467 w1472]
            tunnel: [w1458 w1466 _] -> w1448
            tunnel: w1431 -> [w1457 w1465 _]
            tunnel: w1438 -> [w1456 w1464 _]
            tunnel: [w1455 w1463 _] -> w1432
            frame "KWP-2000" {
              n442 = call <vilib>:"StartRoutineByLocalIdentifier.vi"("error in (no error)"=w1459, "data in"=w1456, "local ID"=w1457, "diag ref in"=w1460) -> ("error out"=w1462:errorcluster, "success?"=w1458:bool, "data out"=w1455:u8[], "diag ref out"=w1461:T29)  [unwired: 4 in]
            }
            frame "UDS" {
              w1470 = u8 1 items=["Start routine"=1, "Stop routine"=2, "Request routine results"=3] ("mode")
              n443 = call <vilib>:"UDS RoutineControl.vi"("mode"=w1470, "error in (no error)"=w1468, "data in"=w1464, "ID"=w1465, "diag ref in"=w1467) -> ("error out"=w1471:errorcluster, "success?"=w1466:bool, "data out"=w1463:u8[], "diag ref out"=w1469:T29)  [unwired: 3 in]
            }
            frame "GMLAN" {
            }
          }
          n444 = call "ScaleAndReplaceAcquiredData.vi"("Lookup"=w1429, "error in (no error)"=w1430, "Unscaled Data"=w1432, "ID"=w1431, "VS Data"=w1428) -> ("error out"=w1427:errorcluster, "VS Data"=w1424:dbl[])  [unwired: 5 in]
          n445 = RT FIFO Write(0:w1426, 1:w1424, 3:w1427) -> (8:w1425:refnum<k33>, 11:w1423:errorcluster)  [unwired: 2 in, 2 out]
          n446 = call "Get Error Byte.vi"("error"=w1423) -> ("error  out"=w1422:errorcluster, "Error Byte"=w1421:u8)  [unwired: 9 in]
          n447 = call "Convert Boolean to DBL Array.vi"("Error Code"=w1421, "Boolean"=w1448) -> ("DBL Array"=w1451:dbl[])  [unwired: 9 in]
          n448 = RT FIFO Write(0:w1450, 1:w1451) -> (8:w1449:refnum<k33>, 11:w1447:errorcluster)  [unwired: 3 in, 2 out]
          n449 = Merge Errors(w1422, w1447) -> (w1446:errorcluster)
          n450 = in-place-cluster #29("Parameters.ChanRefs.ToVS.Status.Write to VS Engine FIFO"=w1449, "Parameters.Properties.CAN.Diagnostic Protocol"=w1453, "Routine.Start.Resp Lookup"=w1429, "Parameters.ChanRefs.ToVS.Routine.Start.Write to VS Engine FIFO"=w1425, "Parameters.ChanRefs.ToVS.Routine.Start.Pairs.Values"=w1424, "ADCS Connection"=w1452, "Routine.Start.Cmd Lookup"=w1433, "Parameters.ChanRefs.FromVS.Routine.Start.Read from VS Engine FIFO"=w1435, "Parameters.ChanRefs.FromVS.Routine.Start.Pairs.Values"=w1434) -> (w1416:T1)
        }
      }
      frame "RequestRoutineStatus" {
        n451 = in-place {
          in-place-border: w1478 -> [w1504]
          in-place-border: [w1505] -> w1476
          in-place-border: w1477 -> [w1502]
          n452 = in-place-cluster #30(w1475) -> ("Parameters.ChanRefs.ToVS.Status.Write to VS Engine FIFO"=w1509:refnum<k33>, "Parameters.Properties.CAN.Diagnostic Protocol"=w1512:T9, "Routine.Status.Resp Lookup"=w1488:variant, "Parameters.ChanRefs.ToVS.Routine.Status.Write to VS Engine FIFO"=w1485:refnum<k33>, "Parameters.ChanRefs.ToVS.Routine.Status.Pairs.Values"=w1487:dbl[], "ADCS Connection"=w1513:T29, "Routine.Status.Cmd Lookup"=w1492:variant, "Parameters.ChanRefs.FromVS.Routine.Status.Read from VS Engine FIFO"=w1495:refnum<k33>, "Parameters.ChanRefs.FromVS.Routine.Status.Pairs.Values"=w1496:dbl[])
          n453 = Unflatten From String(type=u16 0, binary string=w1502, error in (no error)=w1504) -> (value=w1490:u16, error out=w1499:errorcluster)  [unwired: 2 in, 1 out]
          n454 = RT FIFO Read(0:w1495, 1:w1496, 3:w1499) -> (8:w1494:refnum<k33>, 9:w1500:dbl[], 11:w1501:errorcluster)  [unwired: 1 in, 2 out]
          n455 = call "IndexAndScaleGeneratedData.vi"("Lookup"=w1492, "error in"=w1501, "ID"=w1490, "VS Data"=w1500) -> ("error out"=w1498:errorcluster, "Data"=w1497:u8[], "VS Data"=w1493:dbl[])  [unwired: 5 in]
          n456 = case shown="\"KWP-2000\"" w1512 {
            tunnel: [w1517 w1529 w1531] -> w1489
            tunnel: [w1514 w1527 w1530] -> w1511
            tunnel: w1498 -> [w1519 w1526 w1531]
            tunnel: w1513 -> [w1518 w1525 w1530]
            tunnel: [w1516 w1524 _] -> w1507
            tunnel: w1490 -> [w1520 w1523 _]
            tunnel: w1497 -> [_ w1522 _]
            tunnel: [w1515 w1521 _] -> w1491
            frame "KWP-2000" {
              n457 = call <vilib>:"RequestRoutineResultsByLocalIdentifier.vi"("error in (no error)"=w1519, "local ID"=w1520, "diag ref in"=w1518) -> ("error out"=w1517:errorcluster, "success?"=w1516:bool, "data out"=w1515:u8[], "diag ref out"=w1514:T29)  [unwired: 5 in]
            }
            frame "UDS" {
              w1528 = u8 3 items=["Start routine"=1, "Stop routine"=2, "Request routine results"=3] ("mode")
              n458 = call <vilib>:"UDS RoutineControl.vi"("mode"=w1528, "error in (no error)"=w1526, "data in"=w1522, "ID"=w1523, "diag ref in"=w1525) -> ("error out"=w1529:errorcluster, "success?"=w1524:bool, "data out"=w1521:u8[], "diag ref out"=w1527:T29)  [unwired: 3 in]
            }
            frame "GMLAN" {
            }
          }
          n459 = call "ScaleAndReplaceAcquiredData.vi"("Lookup"=w1488, "error in (no error)"=w1489, "Unscaled Data"=w1491, "ID"=w1490, "VS Data"=w1487) -> ("error out"=w1486:errorcluster, "VS Data"=w1483:dbl[])  [unwired: 5 in]
          n460 = RT FIFO Write(0:w1485, 1:w1483, 3:w1486) -> (8:w1484:refnum<k33>, 11:w1482:errorcluster)  [unwired: 2 in, 2 out]
          n461 = call "Get Error Byte.vi"("error"=w1482) -> ("error  out"=w1481:errorcluster, "Error Byte"=w1480:u8)  [unwired: 9 in]
          n462 = call "Convert Boolean to DBL Array.vi"("Error Code"=w1480, "Boolean"=w1507) -> ("DBL Array"=w1510:dbl[])  [unwired: 9 in]
          n463 = RT FIFO Write(0:w1509, 1:w1510) -> (8:w1508:refnum<k33>, 11:w1506:errorcluster)  [unwired: 3 in, 2 out]
          n464 = Merge Errors(w1481, w1506) -> (w1505:errorcluster)
          n465 = in-place-cluster #30("Parameters.ChanRefs.ToVS.Status.Write to VS Engine FIFO"=w1508, "Parameters.Properties.CAN.Diagnostic Protocol"=w1512, "Routine.Status.Resp Lookup"=w1488, "Parameters.ChanRefs.ToVS.Routine.Status.Write to VS Engine FIFO"=w1484, "Parameters.ChanRefs.ToVS.Routine.Status.Pairs.Values"=w1483, "ADCS Connection"=w1511, "Routine.Status.Cmd Lookup"=w1492, "Parameters.ChanRefs.FromVS.Routine.Status.Read from VS Engine FIFO"=w1494, "Parameters.ChanRefs.FromVS.Routine.Status.Pairs.Values"=w1493) -> (w1474:T1)
        }
      }
      frame "StopRoutine" {
        n466 = in-place {
          in-place-border: w1535 -> [w1562]
          in-place-border: [w1563] -> w1532
          in-place-border: w1534 -> [w1560]
          n467 = in-place-cluster #31(w1536) -> ("Parameters.ChanRefs.ToVS.Status.Write to VS Engine FIFO"=w1567:refnum<k33>, "Parameters.Properties.CAN.Diagnostic Protocol"=w1570:T9, "Routine.Stop.Resp Lookup"=w1546:variant, "Parameters.ChanRefs.ToVS.Routine.Stop.Write to VS Engine FIFO"=w1543:refnum<k33>, "Parameters.ChanRefs.ToVS.Routine.Stop.Pairs.Values"=w1545:dbl[], "ADCS Connection"=w1571:T29, "Routine.Stop.Cmd Lookup"=w1550:variant, "Parameters.ChanRefs.FromVS.Routine.Stop.Read from VS Engine FIFO"=w1553:refnum<k33>, "Parameters.ChanRefs.FromVS.Routine.Stop.Pairs.Values"=w1554:dbl[])
          n468 = Unflatten From String(type=u16 0, binary string=w1560, error in (no error)=w1562) -> (value=w1548:u16, error out=w1557:errorcluster)  [unwired: 2 in, 1 out]
          n469 = RT FIFO Read(0:w1553, 1:w1554, 3:w1557) -> (8:w1552:refnum<k33>, 9:w1558:dbl[], 11:w1559:errorcluster)  [unwired: 1 in, 2 out]
          n470 = call "IndexAndScaleGeneratedData.vi"("Lookup"=w1550, "error in"=w1559, "ID"=w1548, "VS Data"=w1558) -> ("error out"=w1556:errorcluster, "Data"=w1555:u8[], "VS Data"=w1551:dbl[])  [unwired: 5 in]
          n471 = case shown="\"UDS\"" w1570 {
            tunnel: [w1575 w1588 w1590] -> w1547
            tunnel: [w1578 w1586 w1589] -> w1569
            tunnel: w1556 -> [w1574 w1585 w1590]
            tunnel: w1571 -> [w1579 w1584 w1589]
            tunnel: [w1576 w1583 _] -> w1565
            tunnel: w1548 -> [w1573 w1582 _]
            tunnel: w1555 -> [w1572 w1581 _]
            tunnel: [w1577 w1580 _] -> w1549
            frame "KWP-2000" {
              n472 = call <vilib>:"StopRoutineByLocalIdentifier.vi"("error in (no error)"=w1574, "data in"=w1572, "local ID"=w1573, "diag ref in"=w1579) -> ("error out"=w1575:errorcluster, "success?"=w1576:bool, "data out"=w1577:u8[], "diag ref out"=w1578:T29)  [unwired: 4 in]
            }
            frame "UDS" {
              w1587 = u8 2 items=["Start routine"=1, "Stop routine"=2, "Request routine results"=3] ("mode")
              n473 = call <vilib>:"UDS RoutineControl.vi"("mode"=w1587, "error in (no error)"=w1585, "data in"=w1581, "ID"=w1582, "diag ref in"=w1584) -> ("error out"=w1588:errorcluster, "success?"=w1583:bool, "data out"=w1580:u8[], "diag ref out"=w1586:T29)  [unwired: 3 in]
            }
            frame "GMLAN" {
            }
          }
          n474 = call "ScaleAndReplaceAcquiredData.vi"("Lookup"=w1546, "error in (no error)"=w1547, "Unscaled Data"=w1549, "ID"=w1548, "VS Data"=w1545) -> ("error out"=w1544:errorcluster, "VS Data"=w1541:dbl[])  [unwired: 5 in]
          n475 = RT FIFO Write(0:w1543, 1:w1541, 3:w1544) -> (8:w1542:refnum<k33>, 11:w1540:errorcluster)  [unwired: 2 in, 2 out]
          n476 = call "Get Error Byte.vi"("error"=w1540) -> ("error  out"=w1539:errorcluster, "Error Byte"=w1538:u8)  [unwired: 9 in]
          n477 = call "Convert Boolean to DBL Array.vi"("Error Code"=w1538, "Boolean"=w1565) -> ("DBL Array"=w1568:dbl[])  [unwired: 9 in]
          n478 = RT FIFO Write(0:w1567, 1:w1568) -> (8:w1566:refnum<k33>, 11:w1564:errorcluster)  [unwired: 3 in, 2 out]
          n479 = Merge Errors(w1539, w1564) -> (w1563:errorcluster)
          n480 = in-place-cluster #31("Parameters.ChanRefs.ToVS.Status.Write to VS Engine FIFO"=w1566, "Parameters.Properties.CAN.Diagnostic Protocol"=w1570, "Routine.Stop.Resp Lookup"=w1546, "Parameters.ChanRefs.ToVS.Routine.Stop.Write to VS Engine FIFO"=w1542, "Parameters.ChanRefs.ToVS.Routine.Stop.Pairs.Values"=w1541, "ADCS Connection"=w1569, "Routine.Stop.Cmd Lookup"=w1550, "Parameters.ChanRefs.FromVS.Routine.Stop.Read from VS Engine FIFO"=w1552, "Parameters.ChanRefs.FromVS.Routine.Stop.Pairs.Values"=w1551) -> (w1533:T1)
        }
      }
    }
    n481 = disable-structure shown="Default" {
      disable-tunnel: w20 -> [w33 w37]
      disable-tunnel: [_ w37] -> w13
      frame condition #0 {
        n482 = case shown="Default" w33 {
          selector: w33 -> [_ w34]
          frame "" {
          }
          frame Default {
            n483 = Concatenate Strings(w34, "Started" ("string")) -> (w36:string)
            n484 = call <vilib>:"NI VeriStand - Print Debug String.vi"("Message"=w36) -> ()  [unwired: 10 in, 1 out]
          }
        }
      }
      frame condition #1 (active) {
      }
    }
    n485 = call "Tester Present.vi"("error in (no error)"=w12, "State Variables in"=w16) -> ("error out"=w26:errorcluster, "State Variables out"=w15:T1)  [unwired: 8 in]
    n486 = call "Global Stop Actions.vi"("Command"=Stop_Global_Commands."Read", "error in (no error)"=w26, "Stop on Error?"=FALSE, "vi reference"=w23) -> ("error out"=w11:errorcluster, "Latched Stop"=w25:bool)  [unwired: 5 in, 1 out]
    n487 = disable-structure shown="DebugRT==TRUE" {
      disable-tunnel: w13 -> [w38 _]
      disable-tunnel: w11 -> [_ _]
      frame condition #0 {
        n488 = case shown="Default" w38 {
          selector: w38 -> [_ w39]
          frame "" {
          }
          frame Default {
            n489 = Concatenate Strings(w39, "Finished" ("string")) -> (w41:string)
            n490 = call <vilib>:"NI VeriStand - Print Debug String.vi"("Message"=w41) -> ()  [unwired: 10 in, 1 out]
          }
        }
      }
      frame condition #1 (active) {
      }
    }
    n491 = call "Report Error to Process.vi"("Error"=w11, "This VI"=w24) -> ()  [unwired: 10 in]
  }
  "error out" <- w8
